vi "UHR-Fleezers Control (fpga) - Leonardo 04-2018 V2.vi"() -> ()   [LabVIEW 2013]
doc: "UHR-Fleezers Instrument Control Code (fpga)"
uses:
  <vilib>/Platform/TimedLoop/XDataNode/timing_clust.ctl
  <vilib>/Platform/TimedLoop/XDataNode/nitl_modes.ctl
  <vilib>/Platform/TimedLoop/XDataNode/wakeup.ctl
  <vilib>/rvi/eio/common/nirviEmuTemplateMethod_errors.vi
  <vilib>/rvi/Emulation/niFpgaSctlEmulationGetInTimedLoop.vi
  <vilib>/rvi/Emulation/niFpgaEmulationReportErrorSimple.vi
  <vilib>/rvi/Emulation/niFpgaGetClockAttributes.vi
  <vilib>/rvi/Emulation/niFpgaCriticalErrorInLSC.vi
  <vilib>/rvi/FIFO/Fifo_Resource/nirvififoEmulationReadFpgaImpl.vi
  <vilib>/rvi/DataTransferAndStorage/Container/Common/niFpgaContainerGetUniqueNameForEmu.vi
  <vilib>/rvi/DataTransferAndStorage/Container/Common/niFpgaContainerExecOnDevCompGetState.vi
  <vilib>/rvi/interface/RandomDataEmulation/nirviRandomDataFPGAFIFO.vi
  <vilib>/rvi/interface/RandomDataEmulation/niFpgaRandomDataHandleErrors.vi
  <vilib>/rvi/eio/common/nirviEmuReportErrorAndStop.vi
  <vilib>/rvi/Emulation/niFpgaProcessEmulError.vi
  <vilib>/rvi/FIFO/Fifo_Resource/nirvififoEmulationWriteFpgaImpl.vi
  <vilib>/Platform/TimedLoop/XDataNode/XDataNode.xnode
  <vilib>/eio/EIOMethodNode/EIOMethodNode.xnode
  <vilib>/eio/EIONode/EIONode.xnode
  <vilib>/rvi/DataTransferAndStorage/Container/XNode/niFpgaContainer.xnode
  <vilib>/rvi/FIFO/Fifo_Resource/nirvififoEmulationRead.vi
  <vilib>/rvi/FIFO/Fifo_Resource/niFpgaFifoEmulationRefIn.vi
  <vilib>/rvi/interface/RandomDataEmulation/nirviRandomDataFpgaReadWriteTemplate.vi
  <vilib>/rvi/FIFO/Fifo_Resource/nirvififoEmulationWrite.vi
  <vilib>/addons/control/pid/fpga.llb/XNode/niFpgaPID.xnode
  <vilib>/Platform/TimedLoop/XDataNode/XDNodeRunTimeDep.lvlib
  <vilib>/rvi/Memory/Memory_Emulation/niFpgaMemoryEmulationRefIn.vi
panel:
  in  "Tab Control 2":T1(tab)
  out "BD1 amplitude 1 out":u16
  out "BD1 amplitude 2 out":u16
  in  "FB output range":cluster{"output low":i16, "output high":i16}={"output low"=0, "output high"=3000}
  in  "FB Gains":T2={"proportional gain (Kc)"=10, "integral gain (Kc*Ts/Ti)"=5, "derivative gain (Kc*Td/Ts)"=0}
  in  "RF synth green feedback max":i16=4000
  in  "RD":bool=TRUE
  in  "Swap F1 and F2":bool
  in  "Scan BD":bool
  in  "Start scan":bool
  in  "OSK Bd 1":bool
  in  "Reset Bd 1":bool
  in  "PMODE":bool=TRUE
  in  "Number Interlace Cycles":u8=2 min=1 max=3
  in  "Interlace Off Parameters":u8=1 min=1 max=3
  in  "Interlace ON/OFF":bool
  out "DIO Relative phase":i16
  in  "Phase count adjustment (DIO)":i16
  in  "+ phase (DIO)":bool
  out "DIO Late Counter":u8
  in  "DIO count 1 (ticks)":u16=400
  in  "DIO count 2 (ticks)":u16=400
  in  "DIO count 3 (ticks)":u16=400
  out "AI2 Y Sum Set 2":i16
  out "AI2 Y Sum Set 1":i16
  in  "FB Setpoint Set 1":i16 min=0 step=1
  in  "FB Reset Set 1":bool
  in  "FB On/Off Set 1":bool
  in  "FB Reset Set 2":bool
  in  "FB On/Off Set 2":bool
  in  "FB Setpoint Set 2":i16 min=0 step=1
  in  "Amp switch delay":u8=5
  in  "RF synth bd controls green":bool
  in  "Phase Trap 2":fxp<+,14,14>
  in  "Phase Trap 1":fxp<+,14,14>
  in  "Phase offset method":u8
  in  "BD 2 Amplitude 1":u16
  in  "BD 1 Amplitude 1":u16
  in  "BD 2 Frequency 1":u64
  in  "BD 1 Frequency 1":u64
  in  "BD 2 Amplitude 2":u16
  in  "BD 1 Amplitude 2":u16
  in  "BD 2 Frequency 2":u64
  in  "BD 1 Frequency 2":u64
  in  "BD 2 Amplitude 3":u16
  in  "BD 1 Amplitude 3":u16
  in  "BD 2 Frequency 3":u64
  in  "BD 1 Frequency 3":u64
  in  "BD 2 Delay (Ticks)":u8 caption="Count(Ticks)"
  in  "Next trap write delay (ticks)":u8 caption="Count(Ticks)"
  out "Random phase generated":fxp<+,14,14>
  in  "RF phase reset before cycles":bool
  in  "Trap 1 osc enable":bool
  in  "N trap osc periods":i16
  in  "Trap osc period (pts)":i16
  in  "Osc traps":bool
  in  "Initiate trap osc":bool
  in  "Ready Write":bool
  in  "Data":i64
  in  "Address 2":u32
  in  "Osc trap cont.":bool
  in  "Trap 2 osc enable":bool
  out "green FB running":bool
  in  "APD 2 AO scale factor":i16=1
  in  "BD 1 Delay (ticks)":u8
  in  "Tab Control":T3(tab)=enum."MCL trap control"
  in  "Set 3":bool
  in  "Set 2":bool=TRUE
  in  "Set 1":bool=TRUE
  in  "Trap Pos to FIFO":bool
  in  "N of AI1 Int Acq Sets":i16=2 min=1 max=3 step=1
  out "AI Late Counter":u8
  in  "ai count":u16=400
  in  "+ phase":bool
  in  "Phase count adjustment":i16
  out "Relative phase":i16
  in  "AI to FIFO":bool
  out "BD1 Frequency Out 1":u64
  out "BD1 Frequency Out 2":u64
  out "Trap Pos FIFO Timeout":u16
  out "Trap AI FIFO Timeout":u16
  in  "Trap FIFO Set Timeout":i32
  in  "Scan freq.  increment":i64
  in  "Scan steps":u64
  in  "Number of scans":u16
  in  "Cycles per step":u64
  in  "Raster setpoint":fxp<+/-,16,1>
  in  "Raster to target force":bool
  out "Actual Scan freq":u64
  in  "Cont. Scan":bool
  out "Scan I":u64
  in  "Abort scan":bool
  out "Scanning":bool
  in  "FB Min frequency":u64
  in  "FB Max Frequency":u64
  in  "Dynamic Force FB (Ronen)":bool
  in  "Trap pos. FB Range":T4={"FB2 output low"=-1.0, "FB2 output high"=0.999969482421875}
  in  "Trap Pos. FB Gains":T5={"proportional gain (Kc)"=0.999969482421875, "integral gain (Kc*Ts/Ti)"=0.999969482421875, "derivative gain (Kc*Td/Ts)"=0.0}
  in  "B factor":fxp<+/-,32,16>
  in  "Negate Diff?":bool
  in  "Diff FB Measurement?":bool
  in  "FB Trig Integrate":u32=1
  out "TTrig?":bool
  in  "TTrig Negate Pos":bool=TRUE
  out "Trap Pos FB Int Signal":fxp<+/-,24,9> format="%.18g"
  out "Trap Pos FB Int-Norm Signal":fxp<+/-,16,1> format="%.16g"
  in  "FPGA TTrig Thresh":i64
  in  "FPGA Trap Trig":bool
  out "Trap Pos FB Action":i64
  in  "Trap Pos. FB Offset Factor":i64
  in  "Trap Pos. FB Mult Factor":i64=2
  in  "Trap Pos. FB Reset":bool
  in  "Trap Pos FB Monitor T1 or T2":bool
  in  "AI1 X Scale":u16
  in  "Trap Pos FB Int Count":u16=100
  in  "Trap Pos FB Negate Action":bool
  out "AI1 X Set 2":fxp<+/-,16,1>
  out "AI1 X Set 1":fxp<+/-,16,1>
  in  "Trap Pos. FB SP":fxp<+/-,16,1>
  in  "Force feedback":bool
  out "TTrig Sig":i64
  out "TTrig Fin Thresh":i64
  in  "1D or 2D Scan?":bool
  in  "Abort scan (MCL)":bool
  in  "MCL Scan Axis":bool
  in  "Cont. Scan (MCL)":bool
  out "Scan I (MCL)":u64
  in  "Number of scans (MCL)":u16
  out "Scanning MCL":bool
  in  "Scan steps (MCL)":u64
  in  "Cycles per step (MCL)":u64
  in  "Scan freq.  increment (MCL)":i16
  in  "Start scan (MCL)":bool
  in  "AO2 (X)":i16
  in  "AO1 (Y)":i16
  out "MCL Late Counter":u8
  in  "MCL count":u32=800
  out "MCL Relative Phase":i16
  in  "Phase count adjustment (MCL)":i16
  in  "+ phase (MCL)":bool
  in  "Lifetime events to read blue":u16=100
  in  "Lifetime read blue fifo":bool
  out "lifetime events in fifo":u16
  out "APD2 int gate":bool
  in  "APD Gate Operating Mode":u8 max=2 step=1
  in  "Invert APD Gate":bool
  in  "APD Gate OFF Count":u16=100
  in  "APD Gate ON Count":u16=300
  out "APD 1 Gate Late Counter":u8
  out "APD 1 Gate Relative Phase":i16
  in  "Phase count adjustment (APD 1 Gate)":i16
  in  "+ phase (APD 1 Gate)":bool
  out "APD 2 Counts 0":u32
  out "APD 2 Counts 1":u32
  out "APD 1 Counts 0":u32
  out "APD 1 Counts 1":u32
  in  "Phase count adjustment (APD 2 Gate)":i16
  out "APD 2 Gate Late Counter":u8
  out "APD 2 Gate Relative Phase":i16
  in  "+ phase (APD 2 Gate)":bool
  out "APD 3 Counts 0":u32
  out "APD 3 Counts 1":u32
  out "APD 3 Gate Late Counter":u8
  in  "Phase count adjustment (APD 3 Gate)":i16
  out "APD 3 Gate Relative Phase":i16
  in  "+ phase (APD 3 Gate)":bool
  out "APD1 int gate":bool
  out "APD3 int gate":bool
  in  "Lifetime timeout APD1":u16=200
  in  "APD to FIFO":bool
  in  "APD Acq Rate Count":u32=20000000
  out "APD Acq Late Counter":u16
  out "APD Acq Relative Phase":i16
  in  "+ phase (APD Acq)":bool
  in  "Phase Count Adjustment (APD Acq)":i16
  in  "APD 1 AO scale factor":i16=1
  out "APD2 out state":bool
  out "APD1 out state":bool
  out "APD Acq Late?":bool
  in  "D3 2":i16
  in  "I3 2":i16=5
  in  "P3 2":i16=10
  in  "Green FB Setpoint 2":i16=250 min=0 step=1
  in  "Green FB Reset 2":bool
  in  "Green Filter Flipper":bool
  in  "Green interlace OFF count":u16=100
  out "GI Relative phase":i16
  in  "Phase count adjustment (GI)":i16
  in  "+ phase (GI)":bool
  in  "Green interlace ON count":u16=300
  out "GI Late Counter":u8
  in  "Invert GI":bool
  in  "Operating Mode":u8 max=2 step=1
  in  "Current Out":u16=30000
  in  "Green int current ON count adj":u32=150
  in  "Green interlace OFF count 2":u32=900
  in  "Green interlace ON count 2":u32=300
  out "GI Late Counter 2":u16
  in  "Green FB Count":u32=1200
  in  "Phase count adjustment (GI) 2":i16=20
  in  "Green FB Setpoint":i16=250 min=0 step=1
  in  "Invert GI 2":bool
  out "GI Relative phase 2":i16
  in  "+ phase (GI) 2":bool
  in  "Phase count adjustment (Green FB)":i16=10
  out "Green Late Counter":u16
  out "Green FB Relative Phase":i16
  in  "+ phase (Green FB)":bool
  out "Green FB Signals":T6
  out "Green FB Sum":i16
  in  "Green FB Gains":T2={"proportional gain (Kc)"=10, "integral gain (Kc*Ts/Ti)"=5, "derivative gain (Kc*Td/Ts)"=0}
  in  "Green FB On/Off":bool
  in  "Green FB Reset":bool
  out "Green FB Late?":bool
  out "GI Late?":bool
  in  "Operating Mode 2":u8=2 max=2 step=1
  in  "Chassis2/Mod4/AO1":u16
  in  "+ phase (RI)":bool
  out "RI Relative phase":i16
  out "RI Late Counter":u8
  in  "Red interlace ON count":u16=300
  in  "Red interlace OFF count":u16=100
  in  "Invert RI":bool
  in  "Red Laser Operating Mode":u8 max=2 step=1
  in  "Phase count adjustment (RI)":i16
  in  "Phase count adjustment (BI D)":i16
  in  "Blue Laser Operating Mode (D)":u8 max=2 step=1
  in  "Invert BI (D)":bool
  in  "Blue interlace OFF count (D)":u16=100
  in  "Blue interlace ON count (D)":u16=300
  out "Blue Late Counter (D)":u8
  out "BI Relative phase (D)":i16
  in  "+ phase (BI D)":bool
  in  "Lifetime to FIFO":bool
  out "lifetime (ticks)":u16
  # "Raster Scan AOD"
  # "1 (X)"
  # "2 (Y)"
  # "IR Intensity Feedback (RF BD 1)"
  # "FB Gains Set 1"
  # "FB output range 1"
  # "IR Intensity Feedback (RF BD 2) -\nonly when using BD 2 for green laser AOM (not trap Y)"
  # "Keep below 4096 (12 bits) to stay within range of RF board. Going over doesn't saturate, it truncates higher bits."
  # "RF phase offset control"
  # "Methods are:\n0 - Default, do nothing at all (no phase offset writes)\n1 - Manual phase adjustment\n2 - Cycle the phase adjustment using the input phase numbers as increment values for each cycle"
  # "False is usual, True is external loop method"
  # "Parameters if using the external RF switching loop"
  # "Parameters if using the usual internal RF switching method"
  # "FB Triggering Excitation Laser"
  # "Trap Pos. FB Gains"
  # "Trap Pos. FB Range"
  # "AO1 (Y)"
  # "2D"
  # "Trap 3"
  # "1D"
  # "AO2 (X)"
  # "Fl Laser"
  # "APD AO for aligning"
  # "Detection Loop"
  # "Green fluorescent laser digital gate interlacing loop"
  # "0 Forced ON\n1 Forced OFF\n2 Interlacing"
  # "ALEX settings:"
  # "Controls for usual IA ME controls green AOM"
  # "Controls for RF synth board controls green AOM"
  # "Green FB Gains"
  # "Red fluorescent laser digital gate interlacing loop"
  # "Detection Loop"
  # "0 Forced ON\n1 Forced OFF\n2 Interlacing"
  # "Analog/FB Control Loop\n(Disabled)"
  # "Digital Control Loop"
  # "Blue laser intensity reading"
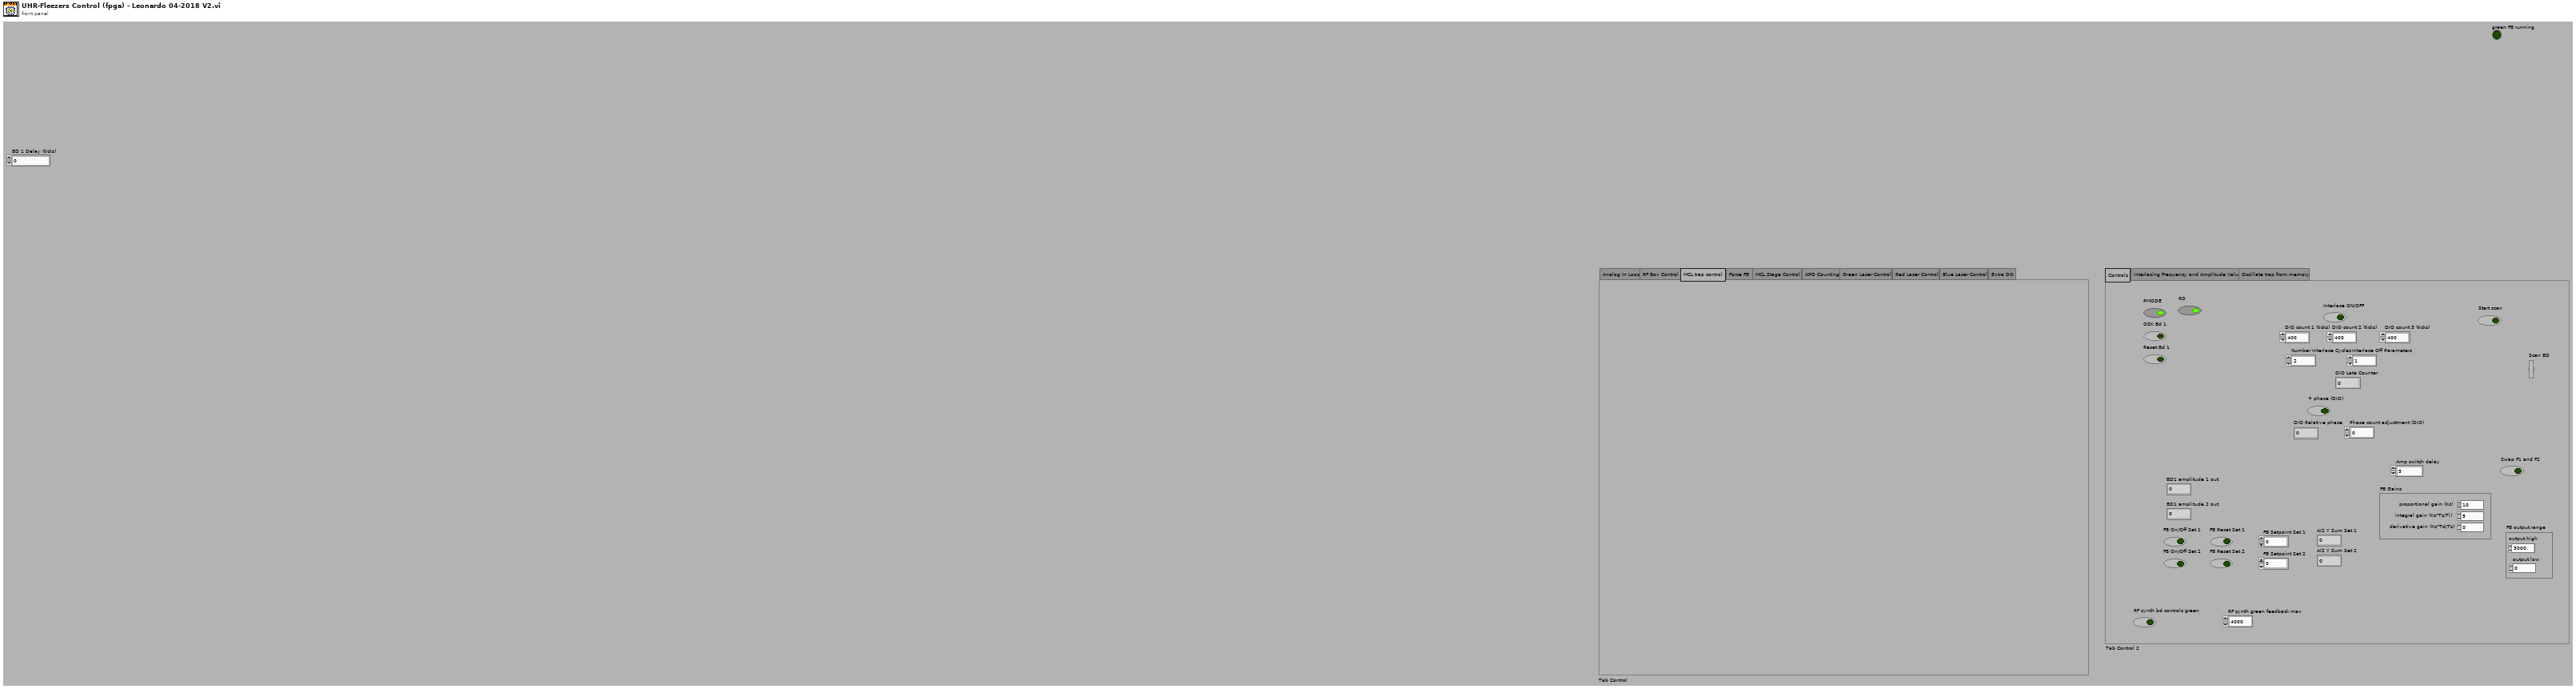
[diagram p1: front panel]
types:
  T1 = enum32{"Controls", "Interlacing Frequency and Amplitude Values", "Oscillate trap from memory"}
  T2 = cluster{"proportional gain (Kc)":i16, "integral gain (Kc*Ts/Ti)":i16, "derivative gain (Kc*Td/Ts)":i16}
  T3 = enum32{"Analog In Loop", "RF Box Control", "MCL trap control", "Force FB", "MCL Stage Control", "APD Counting", "Green Laser Control", "Red Laser Control", "Blue Laser Control", "Extra DO"}
  T4 = cluster{"FB2 output low":fxp<+/-,16,1>, "FB2 output high":fxp<+/-,16,1>}
  T5 = cluster{"proportional gain (Kc)":fxp<+/-,16,1>, "integral gain (Kc*Ts/Ti)":fxp<+/-,16,1>, "derivative gain (Kc*Td/Ts)":fxp<+/-,16,1>}
  T6 = cluster{"Green FB Ch 0":i16, "Green FB Ch 1":i16, "Green FB Ch 2":i16}
  T7 = typedef "XDNodeRunTimeDep.lvlib/timing_clust.ctl" = cluster{"Expected End [f-1]":u64, "Actual End [f-1]":u64, "Finished Late? [f-1]":bool, "Expected End [i-1]":u64, "Actual End [i-1]":u64, "Finished Late? [i-1]":bool, "Expected Start [i]":u64, "Actual Start [i]":u64, "Expected Start [f]":u64, "Actual Start [f]":u64, "Source Name":string, "Structure Name":string, "Period":i64, "Deadline":i64, "Offset":i64, "Start":i64, "Priority":i32, "Timeout":i32, "Mode":T8, "Wakeup Reason":T9, "Error":errorcluster, "Source Type":string, "Secondary Source Type":string, "Global End Time":u64, "Global Start Time":u64, "Frame Duration":u64, "Iteration Duration":u64, "Assigned CPU":i32, "I/O Scan Engine Mode":u32}
  T8 = typedef "XDNodeRunTimeDep.lvlib/nitl_modes.ctl" = enum32{"No Change", "Process missed periods, maintain original phase", "Discard missed periods, maintain original phase", "Process missed periods, ignore original phase", "Discard missed periods, ignore original phase"}
  T9 = typedef "XDNodeRunTimeDep.lvlib/wakeup.ctl" = enum32{"Normal", "Aborted", "Asynchronous wakeup", "Timing source error", "Timed loop error", "Timeout"}
  T10 = cluster{"Chassis2/Mod2/AI0":i16, "Chassis2/Mod2/AI1":i16, "Chassis2/Mod2/AI2":i16}
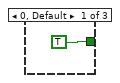
[diagram p3: hidden frame]
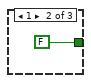
[diagram p4: hidden frame]
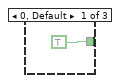
[diagram p8: hidden frame]
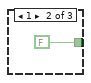
[diagram p9: hidden frame]
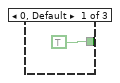
[diagram p10: hidden frame]
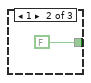
[diagram p11: hidden frame]
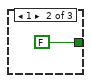
[diagram p13: hidden frame]
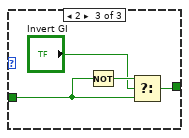
[diagram p14: hidden frame]
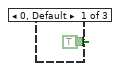
[diagram p15: hidden frame]
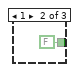
[diagram p16: hidden frame]
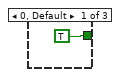
[diagram p18: hidden frame]
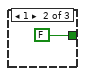
[diagram p19: hidden frame]
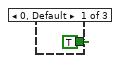
[diagram p20: hidden frame]
diagram:
  w3 = FALSE
  w4 = FALSE
  # "BD2 amp"
  # "BD1 amp"
  # "BD2 amp"
  # "BD1 amp"
  # "timing array current index"
  # "timing array"
  # "timing counter (phase adjusted here)"
  # "late counter"
  n1 = while {
    stop <- FALSE stop-if-true
    n2 = xnode "FPGA I/O Node"("Connector0/DIO3"="Green Filter Flipper", "Chassis2/Mod1/AO1"="Chassis2/Mod4/AO1") -> ()  [unwired: 2 in, 2 out]
    n3 = call "Loop Timer11"("Count(Ticks)"=u32 40000 ("Extra DO Counts")) -> ()  [unwired: 1 out]
  }
  n4 = disable-structure shown="Disabled" {
    frame Disabled {
      w18 = i16 2 items=["UnSet Ready", "ReadWrite", "Wait Ready"]
      n5 = while "Handshake memory transfer for trap oscillation sin wave data" {
        shift-right: [w20] -> _
        shift-left: w18 -> [w21]
        stop <- FALSE stop-if-true
        # "Write"
        n6 = case shown="1" w21 {
          tunnel: [w24 w29 w30] -> w20
          frame 3, Default {
            w22 = i16 2 items=["UnSet Ready", "ReadWrite", "Wait Ready"]
            w23 = i16 1 items=["UnSet Ready", "ReadWrite", "Wait Ready"]
            n7 = Select(t=w23, s="Ready Write", f=w22) -> (s? t:f=w24:i16)
          }
          frame 1 {
            w29 = i16 0 items=["UnSet Ready", "ReadWrite", "Wait Ready"]
            n8 = xnode ("Memory Write")("Address"="Address 2", "Data"="Data", "Memory In"=refnum<k21> "Trap osc memory") -> ()  [unwired: 1 out]
          }
          frame 0 {
            w30 = i16 2 items=["UnSet Ready", "ReadWrite", "Wait Ready"]
            n9 = local write "Ready Write"(FALSE ("Ready Read")) -> ()
          }
        }
      }
    }
    frame Enabled {
    }
  }
  n10 = flat-sequence "FPGA initialization to do before running any of the loops" {
    tunnel: [u16 0 ("DIO count 3 (ticks)")] -> w2
    tunnel: [w39] -> _
    frame #0 {
      # "UDCLK out enable and set low"
      # "WR"
      # "BD 2"
      # "BD 1"
      # "With the RF synth board initialization now done in a separate fpga vi, now when this vi is started, board is already configured and is ready for interlacing. Just need to set WR high and enabled UDCLK as write and set to low.\nbefore setting data and address bits."
      # "Start up expansion chassis early\nto avoid delays later"
      # "Set data and address values to something safe (a correct setting) so any initial WR and udclk flipping doesn't have a chance to mess anything up. Safe would be setting an unused data entry:"
      n11 = xnode "FPGA I/O Method Node"("Enable"=TRUE) -> ("FPGA I/O Out"=w33:refnum<k21>)  [unwired: 1 in]
      n12 = xnode "FPGA I/O Method Node"("Enable"=TRUE) -> ("FPGA I/O Out"=w36:refnum<k21>)  [unwired: 1 in]
      n13 = xnode "FPGA I/O Node"("Chassis2/Mod1/AO0"=u16 0 ("Chassis2/Mod4/AO0")) -> ("Chassis2/Mod2/AI0"=w39:i16)  [unwired: 2 in, 2 out]
      n14 = xnode "FPGA I/O Node"("Connector1/DIO15"=TRUE) -> ()  [unwired: 1 in, 1 out]
      n15 = xnode "FPGA I/O Node"("I/O Item"=FALSE ("Connector1/DIO30"), "FPGA I/O In"=w33) -> ()  [unwired: 1 out]
      n16 = xnode "FPGA I/O Node"("I/O Item"=FALSE ("Connector1/DIO30"), "FPGA I/O In"=w36) -> ()  [unwired: 1 out]
      n17 = xnode "FPGA I/O Node"("Connector1/DIO0"=FALSE, "Connector1/DIO1"=FALSE, "Connector1/DIO2"=FALSE, "Connector1/DIO3"=FALSE, "Connector1/DIO4"=FALSE, "Connector1/DIO5"=FALSE, "Connector1/DIO6"=FALSE, "Connector1/DIO7"=FALSE, "Connector1/DIO8"=FALSE, "Connector1/DIO9"=FALSE, "Connector1/DIO10"=FALSE, "Connector1/DIO11"=FALSE, "Connector1/DIO12"=FALSE, "Connector1/DIO13"=FALSE, "Connector1/DIO20"=FALSE, "Connector1/DIO21"=FALSE, "Connector1/DIO22"=FALSE, "Connector1/DIO23"=FALSE, "Connector1/DIO24"=FALSE, "Connector1/DIO25"=FALSE, "Connector1/DIO26"=FALSE, "Connector1/DIO27"=FALSE, "Connector1/DIO14"=FALSE) -> ()  [unwired: 23 in, 23 out]
    }
  }
  n18 = node-c288() -> (w10:T7)  [unwired: 1 in]
  n19 = timed-loop "RF box board DIO control: control bits" {
    timing: w10 -> [_]
    timing-out: [_] -> w9
    tunnel: [w66] -> _
    tunnel: w2 -> [w66]
    stop <- FALSE stop-if-true
    n20 = xnode "FPGA I/O Node"("Connector1/DIO16"="RD", "Connector1/DIO17"="PMODE", "Connector1/DIO18"="OSK Bd 1", "Connector1/DIO19"="Reset Bd 1") -> ()  [unwired: 4 in, 4 out]
  }
  n21 = node-c288(w9) -> ()
  n22 = local read "AO1 (Y)"() -> (w12:i16)
  n23 = local read "AO2 (X)"() -> (w11:i16)
  n24 = To Unsigned Long Integer(number=w2) -> (unsigned 32bit integer=w5:u32)
  n25 = while "DAQ AI set 1" {
    shift-right: [w73] -> _
    shift-left: w2 -> [w78]
    stop <- FALSE stop-if-true
    n26 = flat-sequence {
      tunnel: w78 -> [w89]
      tunnel: [w88] -> w76
      tunnel: [w89] -> w75
      tunnel: [w99] -> w86
      tunnel: [w98] -> w85
      tunnel: [w97] -> w84
      tunnel: [w96] -> w83
      tunnel: [w95] -> w82
      tunnel: [w94] -> w81
      tunnel: [w93] -> w80
      tunnel: [w92] -> w79
      tunnel: [w91] -> w77
      tunnel: w76 -> [w91]
      tunnel: w75 -> [w90]
      tunnel: [w90] -> w74
      tunnel: [w129] -> w73
      tunnel: w86 -> [w155]
      tunnel: w85 -> [w121]
      tunnel: w84 -> [w122]
      tunnel: w83 -> [w101]
      tunnel: w82 -> [w145]
      tunnel: w81 -> [w144]
      tunnel: w80 -> [w143]
      tunnel: w79 -> [w142]
      tunnel: w77 -> [w139]
      tunnel: w74 -> [w136]
      frame #0 {
        n27 = call "Loop Timer"("Count(Ticks)"=w89) -> ("Tick Count(Ticks)"=w88:u32)
      }
      frame #1 {
        n28 = xnode "FPGA I/O Node"("Connector1/DIO31"=TRUE ("Connector1/DIO33")) -> ("Connector0/AI0"=w99:i16, "Connector0/AI1"=w98:i16, "Connector0/AI2"=w97:i16, "Connector0/AI3"=w96:i16, "Connector0/AI4"=w95:i16, "Connector0/AI5"=w94:i16, "Connector0/AI6"=w93:i16, "Connector0/AI7"=w92:i16)  [unwired: 9 in, 9 out]
      }
      frame #2 {
        w125 = FALSE ("AI to FIFO")
        # "Normalize by trap bead QPD sum, AI3"
        # "Adjust phase after data acquired if button pressed"
        n29 = feedback #1(i16 1) -> (w148:i16)
        n30 = Increment(x=w148) -> (x+1=w154:i16)
        n31 = Scale By Power Of 2(n="AI1 X Scale", x=w121) -> (x*2^n=w119:i16)
        n32 = Greater?(x=w154, y="N of AI1 Int Acq Sets") -> (0:w151:bool)
        n33 = Select(t=i16 1, s=w151, f=w154) -> (s? t:f=w153:i16)
        n34 = feedback-in #1(w153) -> ()
        n35 = Divide(x=w119, y=w101) -> (x/y=w118:fxp<+/-,16,1>)
        n36 = feedback #2(w125) -> (w123:bool)
        n37 = feedback #3(w125) -> (w141:bool)
        n38 = case shown="1, Default" w148 {
          tunnel: w122 -> [w178 w185 _]
          tunnel: ["Set 1" "Set 2" "Set 3"] -> w146
          tunnel: ["AI to FIFO" w187 w192] -> w140
          tunnel: w141 -> [_ w187 w192]
          tunnel: ["Trap Pos to FIFO" w186 w191] -> w124
          tunnel: w123 -> [_ w186 w191]
          tunnel: w118 -> [w177 w184 _]
          tunnel: [w176 w182 FALSE] -> w105
          tunnel: [w175 w183 u64 0 ("BD1 Frequency Out 2")] -> w104
          frame 1, Default {
            n39 = local read "BD1 Frequency Out 1"() -> (w175:u64)
            n40 = Compound Arithmetic op=AND("Trap Pos to FIFO", "Set 1", "AI to FIFO") -> (w176:bool)
            "AI2 Y Sum Set 1" <- w178
            "AI1 X Set 1" <- w177
          }
          frame 2 {
            n41 = local read "BD1 Frequency Out 2"() -> (w183:u64)
            n42 = Compound Arithmetic op=AND(w186, "Set 2", w187) -> (w182:bool)
            "AI2 Y Sum Set 2" <- w185
            "AI1 X Set 2" <- w184
          }
          frame 3 {
          }
        }
        n43 = And(x=w146, y=w140) -> (x .and. y?=w147:bool)
        n44 = case shown="True" w147 {
          tunnel: w155 -> [_ w206]
          tunnel: w121 -> [_ w205]
          tunnel: w122 -> [_ w204]
          tunnel: w101 -> [_ w203]
          tunnel: w145 -> [_ w202]
          tunnel: w144 -> [_ w201]
          tunnel: w143 -> [_ w200]
          tunnel: w142 -> [_ w199]
          tunnel: 0 ("DMA buffer timeout") -> [_ w208]
          frame False {
          }
          frame True {
            n45 = Build Array(w206, w205, w204, w203, w202, w201, w200, w199) -> (w207:i16[])
            n46 = for {
              tunnel: w207 -> [w210] mode=indexing
              tunnel: w208 -> [w211]
              tunnel: [w209] -> w197 mode=indexing
              n47 = xnode ("FIFO Write")("Element"=w210, "Timeout"=w211) -> ("Timed Out?"=w209:bool)  [unwired: 1 in, 1 out]
            }
            n48 = Or Array Elements(Boolean array=w197) -> (logical OR=w194:bool)
            n49 = Boolean To (0,1)(Boolean=w194) -> (0, 1=w196:i16)
            n50 = feedback #4(u16 0) -> (w195:u16)
            n51 = Add(x=w196, y=w195) -> (x+y=w193:u16)
            "Trap AI FIFO Timeout" <- w193
            n52 = feedback-in #4(w193) -> ()
          }
        }
        n53 = feedback-in #2(w124) -> ()
        n54 = feedback-in #3(w140) -> ()
        n55 = case shown="True" w105 {
          tunnel: w104 -> [_ w161]
          tunnel: [u8 0 w158] -> w103
          frame False {
          }
          frame True {
            n56 = Split Number(x=w161) -> (hi(x)=w162:u32, lo(x)=w163:u32)
            n57 = Split Number(x=w162) -> (lo(x)=w164:u16)  [unwired: 1 out]
            n58 = Split Number(x=w163) -> (hi(x)=w165:u16, lo(x)=w166:u16)
            n59 = Build Array "BD 1 nu Stack"(w164, w165, w166) -> (w160:u16[])
            n60 = for {
              tunnel: w160 -> [w173] mode=indexing
              shift-right: [w169] -> w158
              shift-left: u8 0 -> [w170]
              n61 = xnode ("FIFO Method Node")("Element"=w173, "Timeout"="Trap FIFO Set Timeout") -> ("Timed Out?"=w172:bool)  [unwired: 1 in, 1 out]
              n62 = Boolean To (0,1)(Boolean=w172) -> (0, 1=w171:i16)
              n63 = To Unsigned Byte Integer(number=w171) -> (unsigned 8bit integer=w168:u8)
              n64 = Add(x=w168, y=w170) -> (x+y=w169:u8)
            }
          }
        }
        n65 = To Unsigned Word Integer(number=w103) -> (unsigned 16bit integer=w102:u16)
        n66 = feedback #5(u16 0) -> (w116:u16)
        n67 = Add(x=w102, y=w116) -> (x+y=w115:u16)
        "Trap Pos FIFO Timeout" <- w115
        n68 = feedback-in #5(w115) -> ()
        n69 = feedback-in #6(w139) -> ()
        n70 = feedback #6(w139) -> (w138:u32)
        n71 = Subtract(x=w139, y=w138) -> (x-y=w137:u32)
        n72 = xnode "FPGA I/O Node"("Connector1/DIO31"=FALSE ("Connector1/DIO34")) -> ()  [unwired: 1 in, 1 out]
        n73 = Subtract(x=w137, y=w136) -> (x-y=w107:u32)
        n74 = Boolean To (0,1)(Boolean="+ phase") -> (0, 1=w132:i16)
        n75 = Multiply(x=w132, y="Phase count adjustment") -> (x*y=w126:i16)
        n76 = Subtract(x="ai count", y=w107) -> (x-y=w130:u32)
        n77 = Number To Boolean Array(number=w107) -> (Boolean array=w108:bool[])
        n78 = feedback #7(i16 0) -> (w128:i16)
        n79 = Add(x=w130, y=w126) -> (x+y=w129:u32)
        n80 = Subtract(x=w128, y=w126) -> (x-y=w127:i16)
        "Relative phase" <- w127
        n81 = feedback-in #7(w127) -> ()
        n82 = Or Array Elements(Boolean array=w108) -> (logical OR=w106:bool)
        n83 = Boolean To (0,1)(Boolean=w106) -> (0, 1=w113:i16)
        n84 = To Unsigned Byte Integer(number=w113) -> (unsigned 8bit integer=w110:u8)
        n85 = feedback #8(u8 0) -> (w111:u8)
        n86 = Add(x=w110, y=w111) -> (x+y=w109:u8)
        "AI Late Counter" <- w109
        n87 = feedback-in #8(w109) -> ()
      }
    }
  }
  n88 = while "MCL stage control" {
    shift-right: [w224] -> _
    shift-left: w2 -> [w227]
    shift-right: [w217] -> _
    shift-left: w12 -> [w214]
    shift-right: [w216] -> _
    shift-left: w11 -> [w212]
    stop <- FALSE stop-if-true
    n89 = flat-sequence {
      tunnel: w227 -> [w230]
      tunnel: [w229] -> w223
      tunnel: [w230] -> w221
      tunnel: [w232] -> w215
      tunnel: w214 -> [w232]
      tunnel: [w231] -> w213
      tunnel: w212 -> [w231]
      tunnel: w223 -> [w236]
      tunnel: [w236] -> w222
      tunnel: w221 -> [w235]
      tunnel: [w235] -> w220
      tunnel: w215 -> [w234]
      tunnel: w213 -> [w233]
      tunnel: w222 -> [w244]
      tunnel: w220 -> [w243]
      tunnel: [w244] -> w226
      tunnel: [w243] -> w225
      tunnel: [w242] -> w219
      tunnel: [w241] -> w218
      tunnel: [w316] -> w224
      tunnel: w226 -> [w323]
      tunnel: w225 -> [w320]
      tunnel: w219 -> [w318]
      tunnel: w218 -> [w317]
      tunnel: [w318] -> w217
      tunnel: [w317] -> w216
      frame #0 {
        n90 = call "Loop Timer3"("Count(Ticks)"=w230) -> ("Tick Count(Ticks)"=w229:u32)
      }
      frame #1 {
        n91 = xnode "FPGA I/O Node"("Connector0/AO1"=w234, "Connector0/AO2"=w233) -> ()  [unwired: 2 in, 2 out]
      }
      frame #2 {
        n92 = local read "Scanning MCL"() -> (w256:bool)
        n93 = Or(x=w256, y="Start scan (MCL)") -> (x .or. y?=w251:bool)
        n94 = Not(x="Abort scan (MCL)") -> (.not. x?=w249:bool)
        n95 = And(x=w249, y=w251) -> (x .and. y?=w248:bool)
        n96 = case "Raster scan" shown="False" w248 {
          tunnel: [w257 w300] -> w253
          tunnel: "Start scan (MCL)" -> [_ w285]
          tunnel: [w257 w261] -> w237
          frame False {
            w257 = i16 0
            n97 = local write "Scanning MCL"(FALSE ("scanning")) -> ()
          }
          frame True {
            w271 = i16 0
            w270 = u64 0
            # "scan incr."
            # "freq. incr. mult."
            # "count steps"
            # "count number of cycles"
            n98 = feedback #9(w270) -> (w297:u64)
            n99 = Select(t=w270, s=w285, f=w297) -> (s? t:f=w299:u64)
            n100 = Increment(x=w299) -> (x+1=w296:u64)
            n101 = Greater?(x="Cycles per step (MCL)", y=w296) -> (0:w280:bool)
            n102 = Select(t=w296, s=w280, f=w270) -> (s? t:f=w295:u64)
            n103 = feedback-in #9(w295) -> ()
            n104 = feedback #10(w270) -> (w294:u64)
            n105 = Select(t=w270, s=w285, f=w294) -> (s? t:f=w289:u64)
            n106 = Increment(x=w289) -> (x+1=w293:u64)
            n107 = Add(x="Scan steps (MCL)", y="Scan steps (MCL)") -> (x+y=w292:u64)
            n108 = Select(t=w289, s=w280, f=w293) -> (s? t:f=w275:u64)
            n109 = Greater?(x=w292, y=w275) -> (0:w274:bool)
            n110 = Select(t=w275, s=w274, f=w270) -> (s? t:f=w290:u64)
            n111 = feedback-in #10(w290) -> ()
            n112 = Equal?(x="Scan steps (MCL)", y=w275) -> (x = y?=w279:bool)
            n113 = Greater?(x="Scan steps (MCL)", y=w289) -> (0:w288:bool)
            n114 = feedback #11(w271) -> (w291:i16)
            n115 = Select(t=w271, s=w285, f=w291) -> (s? t:f=w277:i16)
            n116 = Increment(x=w277) -> (x+1=w287:i16)
            n117 = Decrement(x=w277) -> (x-1=w286:i16)
            n118 = Select(t=w287, s=w288, f=w286) -> (s? t:f=w278:i16)
            n119 = Select(t=w277, s=w279, f=w278) -> (s? t:f=w276:i16)
            n120 = Select(t=w277, s=w280, f=w276) -> (s? t:f=w272:i16)
            n121 = Select(t=w272, s=w274, f=w271) -> (s? t:f=w273:i16)
            n122 = feedback-in #11(w273) -> ()
            n123 = feedback #12(w270) -> (w284:u64)
            n124 = Select(t=w270, s=w285, f=w284) -> (s? t:f=w259:u64)
            n125 = Increment(x=w259) -> (x+1=w281:u64)
            n126 = Select(t=w259, s=w274, f=w281) -> (s? t:f=w260:u64)
            n127 = Greater?(x="Number of scans (MCL)", y=w260) -> (0:w267:bool)
            n128 = Multiply(x="Scan freq.  increment (MCL)", y=w277) -> (x*y=w300:i16)
            n129 = Select(t=TRUE, s="Cont. Scan (MCL)", f=w267) -> (s? t:f=w266:bool)
            "Scanning MCL" <- w266
            n130 = Select(t=w260, s=w266, f=w270) -> (s? t:f=w282:u64)
            n131 = feedback-in #12(w282) -> ()
            n132 = Increment(x=w260) -> (x+1=→"Scan I (MCL)":u64)
            n133 = To Word Integer(number=w259) -> (16bit integer=w262:i16)
            n134 = Multiply(x=w262, y="Scan freq.  increment (MCL)") -> (x*y=w261:i16)
          }
        }
        n135 = Select(t=w237, s="1D or 2D Scan?", f=i16 0) -> (s? t:f=w238:i16)
        n136 = Select(t=w253, s="MCL Scan Axis", f=w238) -> (s? t:f=w254:i16)
        n137 = Select(t=w238, s="MCL Scan Axis", f=w253) -> (s? t:f=w252:i16)
        n138 = Add(x="AO2 (X)", y=w252) -> (x+y=w241:i16)
        n139 = Add(x="AO1 (Y)", y=w254) -> (x+y=w242:i16)
      }
      frame #3 {
        n140 = feedback-in #13(w323) -> ()
        n141 = feedback #13(w323) -> (w322:u32)
        n142 = Boolean To (0,1)(Boolean="+ phase (MCL)") -> (0, 1=w314:i16)
        n143 = Subtract(x=w323, y=w322) -> (x-y=w321:u32)
        n144 = Multiply(x=w314, y="Phase count adjustment (MCL)") -> (x*y=w310:i16)
        n145 = Subtract(x=w321, y=w320) -> (x-y=w302:u32)
        n146 = Subtract(x="MCL count", y=w302) -> (x-y=w312:u32)
        n147 = feedback #14(i16 0) -> (w311:i16)
        n148 = Subtract(x=w311, y=w310) -> (x-y=w309:i16)
        "MCL Relative Phase" <- w309
        n149 = feedback-in #14(w309) -> ()
        n150 = Number To Boolean Array(number=w302) -> (Boolean array=w303:bool[])
        n151 = Or Array Elements(Boolean array=w303) -> (logical OR=w301:bool)
        n152 = Boolean To (0,1)(Boolean=w301) -> (0, 1=w308:i16)
        n153 = Add(x=w312, y=w310) -> (x+y=w316:u32)
        n154 = To Unsigned Byte Integer(number=w308) -> (unsigned 8bit integer=w305:u8)
        n155 = feedback #15(u8 0) -> (w306:u8)
        n156 = Add(x=w305, y=w306) -> (x+y=w304:u8)
        "MCL Late Counter" <- w304
        n157 = feedback-in #15(w304) -> ()
      }
    }
  }
  n158 = while "APD 2 Counter" {
    tunnel: w2 -> [_]
    stop <- FALSE stop-if-true
    n159 = flat-sequence {
      frame #0 {
        n160 = xnode "FPGA I/O Method Node"("FPGA I/O In"=refnum<k21> "Connector0/DIO1" ("APD 2 DO"), "Timeout"=-1) -> ()  [unwired: 2 out]
      }
      frame #1 {
        n161 = local read "APD2 int gate"() -> (w328:bool)
        n162 = case shown="True" w328 {
          frame False {
          }
          frame True {
            n163 = local read "APD2 out state"() -> (w329:bool)
            n164 = case shown="True" w329 {
              frame False {
                n165 = local read "APD 2 Counts 0"() -> (w331:u32)
                n166 = Increment(x=w331) -> (x+1=→"APD 2 Counts 0":u32)
              }
              frame True {
                n167 = local read "APD 2 Counts 1"() -> (w333:u32)
                n168 = Increment(x=w333) -> (x+1=→"APD 2 Counts 1":u32)
              }
            }
          }
        }
      }
    }
  }
  n169 = while "Green fluorescent laser interlacing (Current to IA 532 nm AOM ME amp)." {
    shift-right: [w339] -> _
    shift-left: w2 -> [w342]
    shift-right: [w336] -> _
    shift-left: i16 0 -> [w334]
    stop <- FALSE stop-if-true
    n170 = flat-sequence {
      tunnel: w342 -> [w345]
      tunnel: [w346] -> w341
      tunnel: [w345] -> w340
      tunnel: [w344] -> w335
      tunnel: w334 -> [w344]
      tunnel: [w349] -> w338
      tunnel: w341 -> [w349]
      tunnel: [w348] -> w337
      tunnel: w340 -> [w348]
      tunnel: w335 -> [w347]
      tunnel: [w362] -> w339
      tunnel: [w378] -> w336
      tunnel: w338 -> [w391]
      tunnel: w337 -> [w388]
      frame #0 {
        n171 = call "Loop Timer10"("Count(Ticks)"=w345) -> ("Tick Count(Ticks)"=w346:u32)
      }
      frame #1 {
        n172 = xnode "FPGA I/O Node"("Chassis2/Mod1/AO0"=w347) -> ()  [unwired: 1 in, 1 out]
      }
      frame #2 {
        n173 = local read "RF synth bd controls green"() -> (w353:bool)
        n174 = Subtract(x="Green interlace OFF count 2", y="Green int current ON count adj") -> (x-y=w371:u32)
        n175 = feedback-in #16(w391) -> ()
        n176 = feedback #16(w391) -> (w390:u32)
        n177 = Add(x="Green int current ON count adj", y="Green interlace ON count 2") -> (x+y=w372:u32)
        n178 = Subtract(x=w391, y=w390) -> (x-y=w389:u32)
        n179 = Subtract(x=w389, y=w388) -> (x-y=w355:u32)
        n180 = Not(x=w353) -> (.not. x?=w351:bool)
        n181 = Number To Boolean Array(number=w355) -> (Boolean array=w356:bool[])
        n182 = Boolean To (0,1)(Boolean="+ phase (GI) 2") -> (0, 1=w368:i16)
        n183 = Or Array Elements(Boolean array=w356) -> (logical OR=w354:bool)
        "GI Late?" <- w354
        n184 = Boolean To (0,1)(Boolean=w354) -> (0, 1=w361:i16)
        n185 = Multiply(x=w368, y="Phase count adjustment (GI) 2") -> (x*y=w364:i16)
        n186 = To Unsigned Word Integer(number=w361) -> (unsigned 16bit integer=w357:u16)
        n187 = feedback #17(u16 0) -> (w359:u16)
        n188 = Add(x=w357, y=w359) -> (x+y=w358:u16)
        "GI Late Counter 2" <- w358
        n189 = feedback-in #17(w358) -> ()
        n190 = feedback #18(i16 0) -> (w365:i16)
        n191 = Subtract(x=w365, y=w364) -> (x-y=w363:i16)
        "GI Relative phase 2" <- w363
        n192 = feedback-in #18(w363) -> ()
        n193 = feedback #19(TRUE) -> (w383:bool)
        n194 = case shown="2" "Operating Mode 2" {
          tunnel: [TRUE FALSE w408] -> w373
          tunnel: w383 -> [_ _ w405]
          frame 0, Default {
          }
          frame 1 {
          }
          frame 2 {
            n195 = Not(x=w405) -> (.not. x?=w407:bool)
            n196 = Select(t=w407, s="Invert GI 2", f=w405) -> (s? t:f=w408:bool)
          }
        }
        n197 = And(x=w373, y="Green FB On/Off") -> (x .and. y?=w352:bool)
        "green FB running" <- w352
        n198 = And(x=w352, y=w351) -> (x .and. y?=w350:bool)
        n199 = case shown="True" w350 {
          tunnel: "Current Out" -> [w392 _]
          tunnel: [w392 w397] -> w377
          frame False {
          }
          frame True {
            n200 = local read "Green FB Sum"() -> (w393:i16)
            n201 = call "Slower PID.vi"("process variable"=w393, "reset?"="Green FB Reset", "setpoint"="Green FB Setpoint", "PID gains (x 2^8)"="Green FB Gains", "output range"=cluster{"output high":i16, "output low":i16} {"output high"=32767, "output low"=-32768} ("Green FB output range")) -> ("output"=w401:i16)  [unwired: 10 out]
            n202 = To Long Integer(number=w401) -> (32bit integer=w394:i32)
            n203 = Add(x=w394, y=32768) -> (x+y=w396:i32)
            n204 = To Unsigned Word Integer(number=w396) -> (unsigned 16bit integer=w397:u16)
          }
        }
        n205 = Not(x=w383) -> (.not. x?=w380:bool)
        n206 = Select(t=w372, s=w380, f=w371) -> (s? t:f=w385:u32)
        n207 = Subtract(x=w385, y=w355) -> (x-y=w366:u32)
        n208 = Add(x=w366, y=w364) -> (x+y=w362:u32)
        n209 = feedback-in #19(w380) -> ()
        n210 = Boolean To (0,1)(Boolean=w373) -> (0, 1=w379:i16)
        n211 = To Unsigned Word Integer(number=w379) -> (unsigned 16bit integer=w376:u16)
        n212 = Multiply(x=w376, y=w377) -> (x*y=w378:u16)
      }
    }
  }
  n213 = while "APD 1 Counter" {
    tunnel: w2 -> [_]
    stop <- FALSE stop-if-true
    n214 = flat-sequence {
      frame #0 {
        n215 = xnode "FPGA I/O Method Node"("FPGA I/O In"=refnum<k21> "Connector0/DIO0" ("APD 1 DO"), "Timeout"=-1) -> ()  [unwired: 2 out]
      }
      frame #1 {
        n216 = local read "APD1 int gate"() -> (w412:bool)
        n217 = case shown="False" w412 {
          frame False {
          }
          frame True {
            n218 = local read "APD1 out state"() -> (w413:bool)
            n219 = case shown="True" w413 {
              frame False {
                n220 = local read "APD 1 Counts 0"() -> (w415:u32)
                n221 = Increment(x=w415) -> (x+1=→"APD 1 Counts 0":u32)
              }
              frame True {
                n222 = local read "APD 1 Counts 1"() -> (w417:u32)
                n223 = Increment(x=w417) -> (x+1=→"APD 1 Counts 1":u32)
              }
            }
          }
        }
      }
    }
  }
  n224 = while "RF synth board interlacing timing loop" {
    tunnel: w2 -> [_]
    stop <- FALSE stop-if-true
    # "This loop is stalled until the RF FIFO get a value. With this method we gain additional delay time (because  we allow the rest of the main RF loop to procede while this loop waits to send the switch signals - a form of parallelism). This helps to simplify the main RF code. \n\nThe code also allow optimal interlacing while also controlling trap RF phase. \n\nNote: a lot of work has gone into optimizing these methods and it is unclear how they can be made any faster or better than this (many failed tries). Right now there is essentially ~4 ticks (~90 ns ns) of imperfection in the switching from trap 1 to trap 2. ~2 ticks of no RF (phase reset) then ~2 ticks of trap 2 with the wrong amplitude (T1 amplitude). The total ticks is 200, so not a big error.\n\nPhase can be precisely set for each trap. Phase reset and switching, has similar delays as fsk frequency switching. And phase reset and phase offset changes are also not simultaneous. So we can't perfectly line everything up.\n\nIf you start from amp zero though (as for trap 1), the on switch is perfect. Likewise the off is perfect for trap 2. \n\nThe green laser switching is also perfect because of its reduced duty cycle and delays in fsk switching between 80 and 0 MHz."
    n225 = xnode ("FIFO Read")("Timeout"=-1) -> ("Element"=w464:u16, "FIFO Out"=w460:refnum<k21>)  [unwired: 1 in, 1 out]
    n226 = Equal To 0?(x=w464) -> (x = 0?=w461:bool)
    n227 = Not(x=w461) -> (.not. x?=w418:bool)
    n228 = flat-sequence "BD 1 and 2 RF phase and amplitude switching" {
      tunnel: w418 -> [_]
      tunnel: w453 -> [w568]
      tunnel: w452 -> [w567]
      tunnel: w451 -> [w566]
      tunnel: w450 -> [w565]
      tunnel: w449 -> [w564]
      tunnel: w448 -> [w563]
      tunnel: w447 -> [w562]
      tunnel: w446 -> [w561]
      tunnel: w444 -> [w560]
      tunnel: w443 -> [w559]
      tunnel: w442 -> [w558]
      tunnel: w440 -> [w556]
      tunnel: w439 -> [w555]
      tunnel: w438 -> [w554]
      tunnel: w441 -> [w557]
      tunnel: w445 -> [w553]
      tunnel: w437 -> [w592]
      tunnel: w436 -> [w591]
      tunnel: w435 -> [w590]
      tunnel: w434 -> [w589]
      tunnel: w433 -> [w588]
      tunnel: w432 -> [w587]
      tunnel: w431 -> [w586]
      tunnel: w430 -> [w585]
      tunnel: w429 -> [w584]
      tunnel: w427 -> [w583]
      tunnel: w426 -> [w582]
      tunnel: w425 -> [w581]
      tunnel: w424 -> [w580]
      tunnel: w423 -> [w579]
      tunnel: w422 -> [w578]
      tunnel: w428 -> [w577]
      frame #0 {
        # "Delay to align amp/frequency switching depending on the method used.\n\nCan also give enough time to do the parallel amplitude calculations"
        n229 = call "Wait2"("Count(Ticks)"="Amp switch delay") -> ()  [unwired: 1 out]
      }
      frame #1 {
        w548 = TRUE ("Connector1/DIO30")
        # "make phase offset and phase reset active with buffer transfer"
        n230 = xnode "FPGA I/O Node"("Connector1/DIO29"=w548, "Connector1/DIO30"=w548) -> ()  [unwired: 2 in, 2 out]
      }
      frame #2 {
        w549 = FALSE ("Connector1/DIO15")
        # "write phase restart to buffer and reset udclk"
        n231 = xnode "FPGA I/O Node"("Connector1/DIO29"=w549, "Connector1/DIO30"=w549, "Connector1/DIO15"=FALSE ("Connector1/DIO14")) -> ()  [unwired: 3 in, 3 out]
      }
      frame #3 {
        w551 = TRUE ("Connector1/DIO15")
        # "make phase restart active"
        # "reset WR"
        n232 = xnode "FPGA I/O Node"("Connector1/DIO15"=w551, "Connector1/DIO29"=w551, "Connector1/DIO30"=w551) -> ()  [unwired: 3 in, 3 out]
      }
      frame #4 {
        w552 = FALSE ("Connector1/DIO30")
        # "Address"
        # "set amp byte 1, and reset udclk"
        n233 = xnode "FPGA I/O Node"("Connector1/DIO0"=w568, "Connector1/DIO1"=w567, "Connector1/DIO2"=w566, "Connector1/DIO3"=w565, "Connector1/DIO4"=w564, "Connector1/DIO5"=w563, "Connector1/DIO6"=w562, "Connector1/DIO7"=w561, "Connector1/DIO8"=TRUE, "Connector1/DIO9"=FALSE, "Connector1/DIO10"=FALSE, "Connector1/DIO11"=FALSE, "Connector1/DIO12"=FALSE, "Connector1/DIO13"=TRUE, "Connector1/DIO20"=w553, "Connector1/DIO21"=w560, "Connector1/DIO22"=w559, "Connector1/DIO23"=w558, "Connector1/DIO24"=w557, "Connector1/DIO25"=w556, "Connector1/DIO26"=w555, "Connector1/DIO27"=w554, "Connector1/DIO30"=w552, "Connector1/DIO29"=w552) -> ()  [unwired: 24 in, 24 out]
      }
      frame #5 {
        # "write amp byte 1 to buffer"
        n234 = xnode "FPGA I/O Node"("Connector1/DIO15"=FALSE ("Connector1/DIO14")) -> ()  [unwired: 1 in, 1 out]
      }
      frame #6 {
        # "reset WR"
        n235 = xnode "FPGA I/O Node"("Connector1/DIO15"=TRUE) -> ()  [unwired: 1 in, 1 out]
      }
      frame #7 {
        # "Address"
        # "set amp byte 2"
        n236 = xnode "FPGA I/O Node"("Connector1/DIO0"=w592, "Connector1/DIO1"=w591, "Connector1/DIO2"=w590, "Connector1/DIO3"=w589, "Connector1/DIO4"=w588, "Connector1/DIO5"=w587, "Connector1/DIO6"=w586, "Connector1/DIO7"=w585, "Connector1/DIO8"=TRUE, "Connector1/DIO9"=FALSE, "Connector1/DIO10"=FALSE, "Connector1/DIO11"=FALSE, "Connector1/DIO12"=TRUE, "Connector1/DIO13"=FALSE, "Connector1/DIO20"=w584, "Connector1/DIO21"=w577, "Connector1/DIO22"=w583, "Connector1/DIO23"=w582, "Connector1/DIO24"=w581, "Connector1/DIO25"=w580, "Connector1/DIO26"=w579, "Connector1/DIO27"=w578) -> ()  [unwired: 22 in, 22 out]
      }
      frame #8 {
        # "write amp byte 2"
        n237 = xnode "FPGA I/O Node"("Connector1/DIO15"=FALSE ("Connector1/DIO14")) -> ()  [unwired: 1 in, 1 out]
      }
      frame #9 {
        w600 = TRUE ("Connector1/DIO15")
        # "transfer amp bytes 1 and 2 and reset WR"
        n238 = xnode "FPGA I/O Node"("Connector1/DIO29"=w600, "Connector1/DIO30"=w600, "Connector1/DIO15"=TRUE ("Connector1/DIO14")) -> ()  [unwired: 3 in, 3 out]
      }
      frame #10 {
        w602 = FALSE ("Connector1/DIO14")
        # "reset udclk"
        n239 = xnode "FPGA I/O Node"("Connector1/DIO29"=w602, "Connector1/DIO30"=w602) -> ()  [unwired: 2 in, 2 out]
      }
    }
    n240 = flat-sequence "FSK BD 1 (trap X)" {
      tunnel: w418 -> [w466]
      tunnel: [w466] -> w421
      tunnel: w421 -> [w467]
      frame #0 {
        n241 = call "Wait"("Count(Ticks)"="BD 1 Delay (ticks)") -> ()  [unwired: 1 out]
      }
      frame #1 {
        # "switch frequency"
        n242 = xnode "FPGA I/O Node"("Connector1/DIO36"=w467) -> ()  [unwired: 1 in, 1 out]
      }
    }
    n243 = flat-sequence "FSK BD 2 (trap Y or green laser AOM)" {
      tunnel: w418 -> [w604]
      tunnel: [w604] -> w463
      tunnel: w463 -> [w605]
      frame #0 {
        n244 = call "Wait3"("Count(Ticks)"="BD 2 Delay (Ticks)") -> ()  [unwired: 1 out]
      }
      frame #1 {
        # "switch frequency"
        n245 = xnode "FPGA I/O Node"("Connector1/DIO37"=w605) -> ()  [unwired: 1 in, 1 out]
      }
    }
    n246 = xnode ("FIFO Read")("Timeout"=-1, "FIFO In"=w460) -> ("Element"=w455:u16, "FIFO Out"=w459:refnum<k21>)  [unwired: 1 out]
    n247 = xnode ("FIFO Read")("Timeout"=-1, "FIFO In"=w459) -> ("Element"=w454:u16)  [unwired: 2 out]
    n248 = node-c288() -> (w457:T7)  [unwired: 1 in]
    n249 = timed-loop "Convert amplitude words to bits" {
      timing: w457 -> [_]
      timing-out: [_] -> w456
      tunnel: w455 -> [w524]
      tunnel: w454 -> [w523]
      tunnel: [w500] -> w453
      tunnel: [w499] -> w452
      tunnel: [w498] -> w451
      tunnel: [w497] -> w450
      tunnel: [w496] -> w449
      tunnel: [w495] -> w448
      tunnel: [w494] -> w447
      tunnel: [w493] -> w446
      tunnel: [w492] -> w445
      tunnel: [w491] -> w444
      tunnel: [w490] -> w443
      tunnel: [w489] -> w442
      tunnel: [w488] -> w441
      tunnel: [w487] -> w440
      tunnel: [w486] -> w439
      tunnel: [w485] -> w438
      tunnel: [w484] -> w437
      tunnel: [w483] -> w436
      tunnel: [w482] -> w435
      tunnel: [w481] -> w434
      tunnel: [w480] -> w433
      tunnel: [w479] -> w432
      tunnel: [w478] -> w431
      tunnel: [w477] -> w430
      tunnel: [w476] -> w429
      tunnel: [w475] -> w428
      tunnel: [w474] -> w427
      tunnel: [w473] -> w426
      tunnel: [w472] -> w425
      tunnel: [w471] -> w424
      tunnel: [w470] -> w423
      tunnel: [w469] -> w422
      stop <- TRUE stop-if-true
      # "Board 1 Data"
      # "Board 2 Data"
      # "Board 1 Data"
      # "Board 2 Data"
      n250 = Split Number(x=w524) -> (hi(x)=w522:u8, lo(x)=w502:u8)
      n251 = Split Number(x=w523) -> (hi(x)=w521:u8, lo(x)=w501:u8)
      n252 = Number To Boolean Array(number=w522) -> (Boolean array=w542:bool[])
      n253 = Number To Boolean Array(number=w521) -> (Boolean array=w533:bool[])
      n254 = Index Array(array=w542, index=7) -> (element=w500:bool)
      n255 = Index Array(array=w542, index=6) -> (element=w499:bool)
      n256 = Index Array(array=w542, index=5) -> (element=w498:bool)
      n257 = Index Array(array=w542, index=4) -> (element=w497:bool)
      n258 = Index Array(array=w542, index=3) -> (element=w496:bool)
      n259 = Index Array(array=w542, index=2) -> (element=w495:bool)
      n260 = Index Array(array=w542, index=1) -> (element=w494:bool)
      n261 = Index Array(array=w542, index=0) -> (element=w493:bool)
      n262 = Index Array(array=w533, index=7) -> (element=w492:bool)
      n263 = Index Array(array=w533, index=6) -> (element=w491:bool)
      n264 = Index Array(array=w533, index=5) -> (element=w490:bool)
      n265 = Index Array(array=w533, index=4) -> (element=w489:bool)
      n266 = Index Array(array=w533, index=3) -> (element=w488:bool)
      n267 = Index Array(array=w533, index=2) -> (element=w487:bool)
      n268 = Index Array(array=w533, index=1) -> (element=w486:bool)
      n269 = Index Array(array=w533, index=0) -> (element=w485:bool)
      n270 = Number To Boolean Array(number=w502) -> (Boolean array=w520:bool[])
      n271 = Number To Boolean Array(number=w501) -> (Boolean array=w511:bool[])
      n272 = Index Array(array=w520, index=7) -> (element=w484:bool)
      n273 = Index Array(array=w520, index=6) -> (element=w483:bool)
      n274 = Index Array(array=w520, index=5) -> (element=w482:bool)
      n275 = Index Array(array=w520, index=4) -> (element=w481:bool)
      n276 = Index Array(array=w520, index=3) -> (element=w480:bool)
      n277 = Index Array(array=w520, index=2) -> (element=w479:bool)
      n278 = Index Array(array=w520, index=1) -> (element=w478:bool)
      n279 = Index Array(array=w520, index=0) -> (element=w477:bool)
      n280 = Index Array(array=w511, index=7) -> (element=w476:bool)
      n281 = Index Array(array=w511, index=6) -> (element=w475:bool)
      n282 = Index Array(array=w511, index=5) -> (element=w474:bool)
      n283 = Index Array(array=w511, index=4) -> (element=w473:bool)
      n284 = Index Array(array=w511, index=3) -> (element=w472:bool)
      n285 = Index Array(array=w511, index=2) -> (element=w471:bool)
      n286 = Index Array(array=w511, index=1) -> (element=w470:bool)
      n287 = Index Array(array=w511, index=0) -> (element=w469:bool)
    }
    n288 = node-c288(w456) -> ()
  }
  n289 = while "APD 1 Gating" {
    shift-right: [w609] -> _
    shift-left: w2 -> [w614]
    shift-right: [w608] -> _
    shift-left: w4 -> [w606]
    stop <- FALSE stop-if-true
    n290 = flat-sequence {
      tunnel: w614 -> [w617]
      tunnel: [w618] -> w612
      tunnel: [w617] -> w610
      tunnel: [w616] -> w607
      tunnel: w606 -> [w616]
      tunnel: [w621] -> w613
      tunnel: w612 -> [w621]
      tunnel: [w620] -> w611
      tunnel: w610 -> [w620]
      tunnel: w607 -> [w619]
      tunnel: [w639] -> w609
      tunnel: w613 -> [w653]
      tunnel: w611 -> [w650]
      tunnel: [w622] -> w608
      frame #0 {
        n291 = call "Loop Timer4"("Count(Ticks)"=w617) -> ("Tick Count(Ticks)"=w618:u32)
      }
      frame #1 {
        # "Signal maybe then sent through \na transistor before APD"
        n292 = xnode "FPGA I/O Node"("Connector1/DIO33"=w619) -> ()  [unwired: 1 in, 1 out]
        "APD1 int gate" <- w619
      }
      frame #2 {
        n293 = feedback #20(TRUE) -> (w645:bool)
        n294 = feedback-in #21(w653) -> ()
        n295 = feedback #21(w653) -> (w652:u32)
        n296 = Not(x=w645) -> (.not. x?=w642:bool)
        n297 = feedback-in #20(w642) -> ()
        n298 = Subtract(x=w653, y=w652) -> (x-y=w651:u32)
        n299 = Select(t="APD Gate ON Count", s=w642, f="APD Gate OFF Count") -> (s? t:f=w647:u16)
        n300 = Subtract(x=w651, y=w650) -> (x-y=w627:u32)
        n301 = Subtract(x=w647, y=w627) -> (x-y=w638:u32)
        n302 = Number To Boolean Array(number=w627) -> (Boolean array=w628:bool[])
        n303 = Or Array Elements(Boolean array=w628) -> (logical OR=w626:bool)
        n304 = Boolean To (0,1)(Boolean="+ phase (APD 1 Gate)") -> (0, 1=w636:i16)
        n305 = Boolean To (0,1)(Boolean=w626) -> (0, 1=w633:i16)
        n306 = Multiply(x=w636, y="Phase count adjustment (APD 1 Gate)") -> (x*y=w634:i16)
        n307 = To Unsigned Byte Integer(number=w633) -> (unsigned 8bit integer=w630:u8)
        n308 = Add(x=w638, y=w634) -> (x+y=w639:u32)
        n309 = feedback #22(i16 0) -> (w641:i16)
        n310 = Subtract(x=w641, y=w634) -> (x-y=w640:i16)
        "APD 1 Gate Relative Phase" <- w640
        n311 = feedback-in #22(w640) -> ()
        n312 = feedback #23(u8 0) -> (w631:u8)
        n313 = Add(x=w630, y=w631) -> (x+y=w629:u8)
        "APD 1 Gate Late Counter" <- w629
        n314 = feedback-in #23(w629) -> ()
        n315 = case shown="2" "APD Gate Operating Mode" {
          tunnel: [TRUE FALSE w656] -> w623
          tunnel: w645 -> [_ _ w656]
          frame 0, Default {
          }
          frame 1 {
          }
          frame 2 {
          }
        }
        n316 = Not(x=w623) -> (.not. x?=w624:bool)
        n317 = Select(t=w624, s="Invert APD Gate", f=w623) -> (s? t:f=w622:bool)
      }
    }
  }
  n318 = while "APD 2 Gating" {
    shift-right: [w660] -> _
    shift-left: w2 -> [w665]
    shift-right: [w659] -> _
    shift-left: w4 -> [w657]
    stop <- FALSE stop-if-true
    n319 = flat-sequence {
      tunnel: w665 -> [w668]
      tunnel: [w669] -> w663
      tunnel: [w668] -> w661
      tunnel: [w667] -> w658
      tunnel: w657 -> [w667]
      tunnel: [w672] -> w664
      tunnel: w663 -> [w672]
      tunnel: [w671] -> w662
      tunnel: w661 -> [w671]
      tunnel: w658 -> [w670]
      tunnel: [w694] -> w660
      tunnel: w664 -> [w704]
      tunnel: w662 -> [w702]
      tunnel: [w673] -> w659
      frame #0 {
        n320 = call "Loop Timer3"("Count(Ticks)"=w668) -> ("Tick Count(Ticks)"=w669:u32)
      }
      frame #1 {
        # "Signal maybe then sent through \na transistor before APD"
        n321 = xnode "FPGA I/O Node"("Connector1/DIO34"=w670) -> ()  [unwired: 1 in, 1 out]
        "APD2 int gate" <- w670
      }
      frame #2 {
        n322 = local read "APD Gate ON Count"() -> (w687:u16)
        n323 = local read "APD Gate OFF Count"() -> (w686:u16)
        n324 = feedback #24(TRUE) -> (w699:bool)
        n325 = feedback-in #25(w704) -> ()
        n326 = feedback #25(w704) -> (w688:u32)
        n327 = Not(x=w699) -> (.not. x?=w697:bool)
        n328 = feedback-in #24(w697) -> ()
        n329 = Subtract(x=w704, y=w688) -> (x-y=w703:u32)
        n330 = Select(t=w687, s=w697, f=w686) -> (s? t:f=w701:u16)
        n331 = Subtract(x=w703, y=w702) -> (x-y=w679:u32)
        n332 = Subtract(x=w701, y=w679) -> (x-y=w693:u32)
        n333 = Number To Boolean Array(number=w679) -> (Boolean array=w678:bool[])
        n334 = Or Array Elements(Boolean array=w678) -> (logical OR=w677:bool)
        n335 = Boolean To (0,1)(Boolean="+ phase (APD 2 Gate)") -> (0, 1=w691:i16)
        n336 = Multiply(x=w691, y="Phase count adjustment (APD 2 Gate)") -> (x*y=w689:i16)
        n337 = Boolean To (0,1)(Boolean=w677) -> (0, 1=w684:i16)
        n338 = Add(x=w693, y=w689) -> (x+y=w694:u32)
        n339 = To Unsigned Byte Integer(number=w684) -> (unsigned 8bit integer=w681:u8)
        n340 = feedback #26(i16 0) -> (w696:i16)
        n341 = Subtract(x=w696, y=w689) -> (x-y=w695:i16)
        "APD 2 Gate Relative Phase" <- w695
        n342 = feedback-in #26(w695) -> ()
        n343 = feedback #27(u8 0) -> (w682:u8)
        n344 = Add(x=w681, y=w682) -> (x+y=w680:u8)
        "APD 2 Gate Late Counter" <- w680
        n345 = feedback-in #27(w680) -> ()
        n346 = local read "APD Gate Operating Mode"() -> (w685:u8)
        n347 = case shown="2" w685 {
          tunnel: [TRUE FALSE w707] -> w674
          tunnel: w699 -> [_ _ w707]
          frame 0, Default {
          }
          frame 1 {
          }
          frame 2 {
          }
        }
        n348 = local read "Invert APD Gate"() -> (w676:bool)
        n349 = Not(x=w674) -> (.not. x?=w675:bool)
        n350 = Select(t=w675, s=w676, f=w674) -> (s? t:f=w673:bool)
      }
    }
  }
  n351 = while "Trap RF control, main calculations (raster scanning, intensity and position feedback, phase control etc) with primary timing trigger" {
    shift-right: [w722] -> _
    shift-left: w2 -> [w721]
    shift-right: [w720] -> _
    shift-left: FALSE ("Swap F1 and F2") -> [w719]
    shift-right: [w715] -> _
    shift-left: u16 0 ("BD 1 Amplitude 3") -> [w712]
    shift-right: [w714] -> _
    shift-left: u16 0 ("BD 2 Amplitude 3") -> [w710]
    shift-right: [w709] -> _
    shift-left: u64 0 -> [w708]
    stop <- FALSE stop-if-true
    n352 = flat-sequence {
      tunnel: w719 -> [w728]
      tunnel: w721 -> [w725]
      tunnel: [w728] -> w718
      tunnel: [w724] -> w717
      tunnel: [w725] -> w716
      tunnel: [w727] -> w713
      tunnel: w712 -> [w727]
      tunnel: [w726] -> w711
      tunnel: w710 -> [w726]
      tunnel: [w739] -> w722
      tunnel: [w738] -> w720
      tunnel: w718 -> [w737]
      tunnel: w717 -> [w736]
      tunnel: w716 -> [w735]
      tunnel: [w734] -> w715
      tunnel: [w733] -> w714
      tunnel: w713 -> [w732]
      tunnel: w711 -> [w731]
      tunnel: [w730] -> w709
      tunnel: w708 -> [w729]
      frame #0 {
        n353 = call "Loop Timer2"("Count(Ticks)"=w725) -> ("Tick Count(Ticks)"=w724:u32)
      }
      frame #1 {
        n354 = flat-sequence {
          tunnel: w737 -> [w747]
          tunnel: w732 -> [w741]
          tunnel: w731 -> [w740]
          tunnel: [w807] -> w739
          tunnel: [w819] -> w738
          tunnel: w736 -> [w813]
          tunnel: w735 -> [w810]
          tunnel: [w758] -> w734
          tunnel: [w757] -> w733
          tunnel: [w749] -> w730
          tunnel: w729 -> [w748]
          frame #0 {
            w742 = -1 ("Timeout")
            # "Operation when you need a long delay for either X or Y to synchonize AOD light out phase (> ~100 ticks)\nor want shorter trap ON timing. Puts some of the delay timing in parallel with the later computations."
            # "Trigger the external loop by sending the boolean FSK value through a FIFO.\nTiming is precise."
            n355 = Boolean To (0,1)(Boolean=w747) -> (0, 1=w746:i16)
            n356 = To Unsigned Word Integer(number=w746) -> (unsigned 16bit integer=w745:u16)
            n357 = xnode ("FIFO Method Node")("Element"=w745, "Timeout"=w742) -> ("FIFO Out"=w744:refnum<k21>)  [unwired: 1 in, 1 out]
            n358 = xnode ("FIFO Method Node")("Element"=w741, "Timeout"=w742, "FIFO In"=w744) -> ("FIFO Out"=w743:refnum<k21>)  [unwired: 1 out]
            n359 = xnode ("FIFO Method Node")("Element"=w740, "Timeout"=w742, "FIFO In"=w743) -> ()  [unwired: 2 out]
          }
          frame #1 {
            # "Just counts, wraps around, 8 bit"
            # "Which trap cycle"
            # "Only save the 3rd set's amp in the loop"
            # "If this is NOT set 3 AND NOT (RF synth controls green AND green FB running)\nthen use this sets amp value (otherwise keep the green feedback value)"
            # "Just flips back and forth."
            # "If interlacing is off, this is which cycle to use."
            # "Keep track of trap cycles (trap 1, 2, 3...)"
            # "This is the prior cycle's on time"
            # "increment timing\nindex, reset to 0 if \nend of matrix"
            # "Reset to begginning (1) when number of cycles reached."
            # "timing index"
            # "build byte stacks for writing data\n(must correspond to addresses array constant)"
            # "Timing housekeeping"
            # "Adjust phase if late\n(maintains constant phase relationship between cycles)"
            n360 = feedback #28(u8 0 ("t")) -> (w816:u8)
            n361 = Increment(x=w816) -> (x+1=w855:u8)
            n362 = Increment(x="Number Interlace Cycles") -> (x+1=w850:u8)
            n363 = Equal?(x=w855, y=w850) -> (x = y?=w857:bool)
            n364 = Select(t=u8 1, s=w857, f=w855) -> (s? t:f=w815:u8)
            n365 = feedback-in #28(w815) -> ()
            n366 = Increment(x=w815) -> (x+1=w852:u8)
            n367 = Equal?(x=w852, y=w850) -> (x = y?=w853:bool)
            n368 = Select "This cycle"(t=u8 1, s=w853, f=w852) -> (s? t:f=w849:u8)
            n369 = Select(t=w849, s="Interlace ON/OFF", f="Interlace Off Parameters") -> (s? t:f=w768:u8)
            n370 = feedback-in #29(w813) -> ()
            n371 = feedback #29(w813) -> (w812:u32)
            n372 = Select(t=w815, s="Interlace ON/OFF", f="Interlace Off Parameters") -> (s? t:f=w848:u8)
            n373 = Subtract(x=w813, y=w812) -> (x-y=w811:u32)
            n374 = Subtract "The error"(x=w811, y=w810) -> (x-y=w794:u32)
            n375 = case shown="1, Default" w848 {
              tunnel: ["DIO count 1 (ticks)" "DIO count 2 (ticks)" "DIO count 3 (ticks)"] -> w809
              frame 1, Default {
              }
              frame 2 {
              }
              frame 3 {
              }
            }
            n376 = Number To Boolean Array(number=w794) -> (Boolean array=w795:bool[])
            n377 = Or Array Elements(Boolean array=w795) -> (logical OR=w793:bool)
            n378 = Boolean To (0,1)(Boolean=w793) -> (0, 1=w800:i16)
            n379 = To Unsigned Byte Integer(number=w800) -> (unsigned 8bit integer=w797:u8)
            n380 = feedback #30(u8 0) -> (w798:u8)
            n381 = Add(x=w797, y=w798) -> (x+y=w796:u8)
            "DIO Late Counter" <- w796
            n382 = feedback-in #30(w796) -> ()
            n383 = Subtract(x=w809, y=w794) -> (x-y=w808:u32)
            n384 = disable-structure shown="Disabled" {
              disable-tunnel: [w861 _] -> w792
              disable-tunnel: w768 -> [w858 _]
              frame Disabled {
                n385 = feedback #31(i64 0 ("y")) -> (w860:i64)
                n386 = case "Synchronize trap oscillations - always begin/end with trap 1" shown="1, Default" w858 {
                  tunnel: [w862 w863 w864] -> w861
                  tunnel: w860 -> [w862 w863 _]
                  frame 2 {
                  }
                  frame 3 {
                  }
                  frame 1, Default {
                    n387 = Or(x="Osc traps", y="Initiate trap osc") -> (x .or. y?=w866:bool)
                    n388 = case "Trap sine oscillation (or whatever pattern is stored in memory)" shown="True" w866 {
                      tunnel: [i64 0 ("y") w870] -> w864
                      tunnel: "Initiate trap osc" -> [_ w873]
                      frame False {
                      }
                      frame True {
                        w877 = u16 0
                        w875 = -1
                        n389 = local write "Initiate trap osc"(FALSE ("Initiate trap osc")) -> ()
                        n390 = feedback #32(w877) -> (w879:u16)
                        n391 = Select(t=w877, s=w873, f=w879) -> (s? t:f=w878:u16)
                        n392 = Greater Or Equal?(x=w878, y="Trap osc period (pts)") -> (x >= y?=w884:bool)
                        n393 = Or(x=w873, y=w884) -> (x .or. y?=w885:bool)
                        n394 = Select(t=u16 0, s=w885, f=w878) -> (s? t:f=w869:u16)
                        n395 = feedback #33(w875) -> (w876:i32)
                        n396 = Select(t=w875, s=w873, f=w876) -> (s? t:f=w874:i32)
                        n397 = Increment(x=w874) -> (x+1=w881:i32)
                        n398 = Equal?(x=w869, y=u16 0) -> (x = y?=w882:bool)
                        n399 = Increment(x=w869) -> (x+1=w889:u16)
                        n400 = feedback-in #32(w889) -> ()
                        n401 = Select(t=w881, s=w882, f=w874) -> (s? t:f=w880:i32)
                        n402 = feedback-in #33(w880) -> ()
                        n403 = case shown="False" "Osc trap cont." {
                          tunnel: w880 -> [w893 _]
                          frame False {
                            n404 = Greater Or Equal?(x=w893, y="N trap osc periods") -> (x >= y?=w891:bool)
                            n405 = Not(x=w891) -> (.not. x?=w890:bool)
                            n406 = local write "Osc traps"(w890) -> ()
                          }
                          frame True {
                          }
                        }
                        n407 = xnode ("Memory Read")("Address"=w869, "Memory In"=refnum<k21> "Trap osc memory") -> ("Data"=w870:i64)  [unwired: 1 out]
                      }
                    }
                  }
                }
                n408 = feedback-in #31(w861) -> ()
              }
              frame Enabled {
              }
            }
            n409 = local read "green FB running"() -> (w781:bool)
            n410 = And(x=w781, y="RF synth bd controls green") -> (x .and. y?=w780:bool)
            n411 = case shown="1, Default" w768 {
              tunnel: [w1020 w1256 "BD 1 Frequency 3"] -> w845
              tunnel: [w1061 w1255 w1277] -> w784
              tunnel: ["BD 2 Amplitude 1" "BD 2 Amplitude 2" w1276] -> w776
              tunnel: [w1017 w1252 "BD 1 Amplitude 3"] -> w758
              tunnel: "FB Gains" -> [w1038 w1262 _]
              tunnel: "FB output range" -> [w1039 w1261 _]
              tunnel: w792 -> [w1036 w1259 _]
              tunnel: "BD 2 Frequency 1" -> [w1033 _ _]
              tunnel: "BD 2 Frequency 2" -> [_ w1255 _]
              tunnel: "BD 2 Frequency 3" -> [_ _ w1277]
              tunnel: w780 -> [_ _ w1275]
              tunnel: [w1020 w1253 w1274] -> w749
              tunnel: w748 -> [w1019 w1253 w1274]
              frame 1, Default {
                w1052 = fxp<+/-,24,9> 0.0 ("AI1 X Set 2")
                w1046 = u16 0
                w1059 = u64 0 ("f")
                # "Changed by Ronen - correction \nby PID is now implemented not on \nthe Base BD1 frequency but on the last\nfrequency sent."
                # "Added by Ronen -\nUpper and Lower \nLimits for the FB \ngenerated frequency\nto avoid losing bead \nwhen tether breaks"
                # "Explanation of raster scanning:\n1. Cycles: increment counter by 1 every time interlace cycle returns to trap 1. As long as \n  Cycle per Step is larger than counter, keep incrementing counter and do not change step counter.\n  Once counter is equal to Cycles per step, zero counter and increment step counter.\n2. Steps: Increments up every time cycles counter equals cycles per step. Performs the following:\n- To determine DIRECTION of frequency change:  If ScanstepX2 is EQUAL to step counter (full for-back scan finished)\n   frequency increment is set to zero, AND step counter is set to zero. \n   Otherwise: if no change to step counter (because cycleperstep>cycle counter), then no change to frequency\n   increment. \n   If step counter has changed (cycleperstep=cycle counter), then need to figure out direction of frequency change:\n   if step counter is EQUAL to Scansteps: No change to frequency increment\n   Otherwise: If scan steps > step counter - 1 (forward scan NOT completed): increment frequency by 1\n                       If scan steps equal or smaller than step counter -1 (forward scan completed): increment frequency by -1\n\n3. Scans: Increment scan counter every time step counter equals 2Xscan steps (full for-back scan completed)\n    if number of scans > scan counter: Send TRUE to scanning, continue scan\n    if number of scans = scan counter: Send FALSE to Scanning, Scan finished.\n\n  The wire with the asterik can be used as the index for getting the mirror positions in the offset scan."
                # "This signal integration happens no matter what\nso that correct setpoints can be chosen before \nturning on the FB."
                # "Trap 1"
                n412 = local read "AI1 X Set 2"() -> (w1031:fxp<+/-,16,1>)
                n413 = local read "AI1 X Set 1"() -> (w1049:fxp<+/-,16,1>)
                n414 = local read "Scanning"() -> (w1062:bool)
                n415 = Multiply(x=w1031, y="B factor") -> (x*y=w1029:fxp<+/-,48,17>)
                n416 = Or(x=w1062, y="Start scan") -> (x .or. y?=w1014:bool)
                n417 = case shown="True" "Diff FB Measurement?" {
                  tunnel: w1029 -> [w1152 w1161]
                  tunnel: w1049 -> [w1151 w1162]
                  tunnel: [w1149 w1153] -> w1050
                  frame False {
                    n418 = Select(t=w1151, s="Trap Pos FB Monitor T1 or T2", f=w1152) -> (s? t:f=w1149:fxp<+/-,48,17>)
                  }
                  frame True {
                    n419 = Subtract(x=w1162, y=w1161) -> (x-y=w1154:fxp<+/-,48,17>)
                    n420 = Not(x="Negate Diff?") -> (.not. x?=w1160:bool)
                    n421 = Boolean To (0,1)(Boolean="Negate Diff?") -> (0, 1=w1158:i16)
                    n422 = Boolean To (0,1)(Boolean=w1160) -> (0, 1=w1159:i16)
                    n423 = Negate(x=w1158) -> (-x=w1157:i16)
                    n424 = Add(x=w1157, y=w1159) -> (x+y=w1155:i16)
                    n425 = Multiply(x=w1155, y=w1154) -> (x*y=w1153:fxp<+/-,63,32>)
                  }
                }
                n426 = feedback #34(w1046) -> (w1045:u16)
                n427 = Increment(x=w1045) -> (x+1=w1047:u16)
                n428 = Greater Or Equal?(x=w1047, y="Trap Pos FB Int Count") -> (x >= y?=w1018:bool)
                n429 = Select(t=w1046, s=w1018, f=w1047) -> (s? t:f=w1048:u16)
                n430 = feedback-in #34(w1048) -> ()
                n431 = feedback #35(w1052) -> (w1051:fxp<+/-,24,9>)
                n432 = Add(x=w1050, y=w1051) -> (x+y=w1044:fxp<+/-,24,9>)
                n433 = Select(t=w1052, s=w1018, f=w1044) -> (s? t:f=w1055:fxp<+/-,24,9>)
                n434 = feedback-in #35(w1055) -> ()
                n435 = case "Trap 1 X intensity feedback" shown="True" "FB On/Off Set 1" {
                  tunnel: "BD 1 Amplitude 1" -> [w1244 _]
                  tunnel: [w1244 w1248] -> w1017
                  tunnel: w1039 -> [_ w1245]
                  tunnel: w1038 -> [_ w1246]
                  frame False {
                  }
                  frame True {
                    n436 = local read "AI2 Y Sum Set 1"() -> (w1249:i16)
                    n437 = call "Slower PID.vi"("process variable"=w1249, "reset?"="FB Reset Set 1", "setpoint"="FB Setpoint Set 1", "PID gains (x 2^8)"=w1246, "output range"=w1245) -> ("output"=w1250:i16)  [unwired: 10 out]
                    n438 = To Unsigned Word Integer(number=w1250) -> (unsigned 16bit integer=w1248:u16)
                  }
                }
                "BD1 amplitude 1 out" <- w1017
                n439 = Divide(x=w1044, y="Trap Pos FB Int Count") -> (x/y=w1015:fxp<+/-,16,1>)
                n440 = case "For raster scanning" shown="True" w1014 {
                  tunnel: [u64 0 w1092] -> w1016
                  tunnel: [FALSE w1080] -> w1009
                  tunnel: [i16 0 w1079] -> w1010
                  tunnel: w1015 -> [_ w1078]
                  tunnel: "Start scan" -> [_ w1072]
                  frame False {
                    n441 = local write "Scanning"(FALSE ("scanning")) -> ()
                  }
                  frame True {
                    w1086 = u64 0
                    # "Changed by RG, to introduce force\ndependent stopping of the raster scan \nand manual stopping"
                    # "count number of cycles"
                    n442 = feedback #36(w1086) -> (w1089:u64)
                    n443 = Select(t=w1086, s=w1072, f=w1089) -> (s? t:f=w1091:u64)
                    n444 = Increment(x=w1091) -> (x+1=w1084:u64)
                    n445 = Equal?(x=i16 1, y=w1084) -> (x = y?=w1082:bool)
                    n446 = And(x="Abort scan", y=w1082) -> (x .and. y?=w1080:bool)
                    n447 = Greater?(x="Cycles per step", y=w1084) -> (0:w1087:bool)
                    n448 = Select(t=w1084, s=w1087, f=w1086) -> (s? t:f=w1088:u64)
                    n449 = feedback-in #36(w1088) -> ()
                    n450 = Greater?(x=w1078, y="Raster setpoint") -> (0:w1075:bool)
                    n451 = And(x=w1075, y="Raster to target force") -> (x .and. y?=w1073:bool)
                    n452 = case shown="False" w1080 {
                      tunnel: [w1099 i16 0] -> w1092
                      tunnel: w1072 -> [w1124 _]
                      tunnel: w1087 -> [w1117 _]
                      tunnel: w1086 -> [w1107 _]
                      tunnel: [w1101 FALSE] -> w1081
                      tunnel: [w1097 w1135] -> w1079
                      tunnel: [w1100 w1136] -> w1076
                      frame False {
                        w1108 = i64 0
                        # "scan incr."
                        # "freq. incr. mult."
                        # "count steps"
                        n453 = feedback #37(w1107) -> (w1132:u64)
                        n454 = Select(t=w1107, s=w1124, f=w1132) -> (s? t:f=w1100:u64)
                        n455 = Increment(x=w1100) -> (x+1=w1131:u64)
                        n456 = Add(x="Scan steps", y="Scan steps") -> (x+y=w1130:u64)
                        n457 = Select(t=w1100, s=w1117, f=w1131) -> (s? t:f=w1112:u64)
                        n458 = Greater?(x=w1130, y=w1112) -> (0:w1111:bool)
                        n459 = Select(t=w1112, s=w1111, f=w1107) -> (s? t:f=w1128:u64)
                        n460 = feedback-in #37(w1128) -> ()
                        n461 = Equal?(x="Scan steps", y=w1112) -> (x = y?=w1116:bool)
                        n462 = Greater?(x="Scan steps", y=w1100) -> (0:w1127:bool)
                        n463 = feedback #38(w1108) -> (w1129:i64)
                        n464 = Select(t=w1108, s=w1124, f=w1129) -> (s? t:f=w1114:i64)
                        n465 = Increment(x=w1114) -> (x+1=w1126:i64)
                        n466 = Decrement(x=w1114) -> (x-1=w1125:i64)
                        n467 = Select(t=w1126, s=w1127, f=w1125) -> (s? t:f=w1115:i64)
                        n468 = Select(t=w1114, s=w1116, f=w1115) -> (s? t:f=w1113:i64)
                        n469 = Select(t=w1114, s=w1117, f=w1113) -> (s? t:f=w1109:i64)
                        n470 = Select(t=w1109, s=w1111, f=w1108) -> (s? t:f=w1110:i64)
                        n471 = feedback-in #38(w1110) -> ()
                        n472 = feedback #39(w1107) -> (w1123:u64)
                        n473 = Select(t=w1107, s=w1124, f=w1123) -> (s? t:f=w1119:u64)
                        n474 = Increment(x=w1119) -> (x+1=w1120:u64)
                        n475 = Select(t=w1119, s=w1111, f=w1120) -> (s? t:f=w1118:u64)
                        n476 = Greater?(x="Number of scans", y=w1118) -> (0:w1104:bool)
                        n477 = Multiply(x="Scan freq.  increment", y=w1114) -> (x*y=w1099:i64)
                        n478 = Select(t=TRUE, s="Cont. Scan", f=w1104) -> (s? t:f=w1101:bool)
                        n479 = Select(t=w1118, s=w1101, f=w1107) -> (s? t:f=w1121:u64)
                        n480 = feedback-in #39(w1121) -> ()
                        n481 = local read "BD 1 Frequency 1"() -> (w1098:u64)
                        n482 = Increment(x=w1118) -> (x+1=→"Scan I":u64)
                        n483 = Add(x=w1099, y=w1098) -> (x+y=w1097:u64)
                        "Actual Scan freq" <- w1097
                      }
                      frame True {
                        n484 = local read "Actual Scan freq"() -> (w1135:u64)
                        n485 = local read "Scan steps"() -> (w1136:u64)
                      }
                    }
                    "Scanning" <- w1081
                    n486 = case shown="True" w1073 {
                      tunnel: w1076 -> [_ w1096]
                      frame False {
                      }
                      frame True {
                        n487 = Add(x=w1096, y=i16 2) -> (x+y=w1094:u64)
                        n488 = local write "Raster to target force"(FALSE) -> ()
                        n489 = local write "Scan steps"(w1094) -> ()
                      }
                    }
                  }
                }
                n490 = feedback #40(fxp<+/-,24,9> 0.0 ("AI1 X Set 2")) -> (w1056:fxp<+/-,24,9>)
                n491 = Select(t=w1044, s=w1018, f=w1056) -> (s? t:f=w1057:fxp<+/-,24,9>)
                "Trap Pos FB Int Signal" <- w1057
                n492 = feedback-in #40(w1057) -> ()
                n493 = feedback #41(fxp<+/-,16,1> 0.0 ("Trap Pos FB Int-Norm Signal")) -> (w1041:fxp<+/-,16,1>)
                n494 = Select(t=w1015, s=w1018, f=w1041) -> (s? t:f=w1040:fxp<+/-,16,1>)
                "Trap Pos FB Int-Norm Signal" <- w1040
                n495 = feedback-in #41(w1040) -> ()
                n496 = case "For position feedback" shown="True" "Force feedback" {
                  tunnel: [i64 0 w1168] -> w1025
                  tunnel: w1015 -> [_ w1165]
                  tunnel: w1018 -> [_ w1164]
                  frame False {
                  }
                  frame True {
                    n497 = feedback #42(i64 0) -> (w1167:i64)
                    n498 = case shown="True" w1164 {
                      tunnel: [w1169 w1173] -> w1168
                      tunnel: w1167 -> [w1169 _]
                      tunnel: w1165 -> [_ w1172]
                      frame False {
                      }
                      frame True {
                        n499 = xnode ("PID")("process variable"=w1172, "reset?"="Trap Pos. FB Reset", "setpoint"="Trap Pos. FB SP", "PID gains"="Trap Pos. FB Gains", "output range"="Trap pos. FB Range") -> ("output"=w1182:fxp<+/-,16,1>)
                        n500 = Negate(x=w1182) -> (-x=w1181:fxp<+/-,17,2>)
                        n501 = Select(t=w1181, s="Trap Pos FB Negate Action", f=w1182) -> (s? t:f=w1178:fxp<+/-,17,2>)
                        n502 = Scale By Power Of 2(n=u32 15, x=u32 1) -> (x*2^n=w1175:u32)
                        n503 = Multiply(x=w1178, y=w1175) -> (x*y=w1174:fxp<+/-,17,17>)
                        n504 = To Quad Integer(1:w1174) -> (0:w1186:i64)
                        "Trap Pos FB Action" <- w1186
                        n505 = Multiply(x=w1186, y="Trap Pos. FB Mult Factor") -> (x*y=w1184:i64)
                        n506 = Add(x=w1184, y="Trap Pos. FB Offset Factor") -> (x+y=w1173:i64)
                        n507 = disable-structure shown="Disabled" {
                          disable-tunnel: w1173 -> [w1193 _]
                          frame Disabled {
                            w1197 = u32 0
                            n508 = feedback #43() -> (w1194:i64)  [unwired: 1 in]
                            n509 = Add(x=w1193, y=w1194) -> (x+y=w1191:i64)
                            n510 = feedback #44(w1197) -> (w1199:u32)
                            n511 = Increment(x=w1199) -> (x+1=w1188:u32)
                            n512 = Greater Or Equal?(x=w1188, y="FB Trig Integrate") -> (x >= y?=w1189:bool)
                            n513 = Select(t=i64 0, s=w1189, f=w1191) -> (s? t:f=w1195:i64)
                            n514 = feedback-in #43(w1195) -> ()
                            n515 = Select(t=w1197, s=w1189, f=w1188) -> (s? t:f=w1198:u32)
                            n516 = feedback-in #44(w1198) -> ()
                            n517 = And(x=w1189, y="FPGA Trap Trig") -> (x .and. y?=w1196:bool)
                            n518 = case "Trap FB trigger excitation laser ON" shown="True" w1196 {
                              tunnel: w1191 -> [_ w1203]
                              tunnel: w1188 -> [_ w1201]
                              frame False {
                              }
                              frame True {
                                n519 = Not(x="TTrig Negate Pos") -> (.not. x?=w1210:bool)
                                n520 = Boolean To (0,1)(Boolean="TTrig Negate Pos") -> (0, 1=w1208:i16)
                                n521 = Boolean To (0,1)(Boolean=w1210) -> (0, 1=w1209:i16)
                                n522 = Negate(x=w1208) -> (-x=w1207:i16)
                                n523 = Add(x=w1207, y=w1209) -> (x+y=w1206:i16)
                                n524 = Multiply(x=w1206, y=w1203) -> (x*y=w1205:i64)
                                "TTrig Sig" <- w1205
                                n525 = Multiply(x="FPGA TTrig Thresh", y=w1201) -> (x*y=w1202:i64)
                                "TTrig Fin Thresh" <- w1202
                                n526 = Greater Or Equal?(x=w1205, y=w1202) -> (x >= y?=w1204:bool)
                                n527 = case shown="True" w1204 {
                                frame False {
                                }
                                frame True {
                                w1213 = TRUE ("Green FB On/Off")
                                w1215 = u8 2 ("Operating Mode")
                                n528 = local write "Operating Mode"(w1215) -> ()
                                n529 = local write item#-1(w1215) -> ()
                                n530 = local write item#-1(w1213) -> ()
                                n531 = local write "FPGA Trap Trig"(FALSE ("FPGA Trap Trig")) -> ()
                                "TTrig?" <- w1213
                                }
                                }
                              }
                            }
                          }
                          frame Enabled {
                          }
                        }
                      }
                    }
                    n532 = feedback-in #42(w1168) -> ()
                  }
                }
                n533 = And(x="Force feedback", y="Dynamic Force FB (Ronen)") -> (x .and. y?=w1026:bool)
                n534 = case shown="True" w1026 {
                  tunnel: w1025 -> [w1140 w1144]
                  tunnel: [w1139 w1143] -> w1011
                  tunnel: w1019 -> [_ w1142]
                  tunnel: w1018 -> [_ w1141]
                  frame False {
                    # "(BD1 Frequency 1)"
                    n535 = Add(x="BD 1 Frequency 1", y=w1140) -> (x+y=w1139:u64)
                  }
                  frame True {
                    n536 = case shown="True" w1141 {
                      tunnel: w1144 -> [_ w1148]
                      tunnel: [w1145 w1147] -> w1143
                      tunnel: w1142 -> [w1145 w1146]
                      frame False {
                      }
                      frame True {
                        n537 = Add(x=w1146, y=w1148) -> (x+y=w1147:u64)
                      }
                    }
                  }
                }
                n538 = case shown="True" w1009 {
                  tunnel: [w1065 w1067] -> w1012
                  tunnel: w1011 -> [w1065 _]
                  tunnel: w1010 -> [_ w1067]
                  frame False {
                  }
                  frame True {
                    n539 = local write "BD 1 Frequency 1"(w1067) -> ()
                    n540 = local write "Abort scan"(FALSE) -> ()
                  }
                }
                n541 = Select(t=w1036, s="Trap 1 osc enable", f=i64 0) -> (s? t:f=w1034:i64)
                n542 = Select(t=w1059, s="Scan BD", f=w1016) -> (s? t:f=w1058:u64)
                n543 = Select(t=w1016, s="Scan BD", f=w1059) -> (s? t:f=w1024:u64)
                n544 = Add(x=w1058, y=w1033) -> (x+y=w1061:u64)
                n545 = Compound Arithmetic op=ADD(w1034, w1012, w1024) -> (w1023:u64)
                n546 = In Range and Coerce(upper limit="FB Max Frequency", x=w1023, lower limit="FB Min frequency") -> (coerced(x)=w1020:u64)  [unwired: 1 out]
                "BD1 Frequency Out 1" <- w1020
              }
              frame 2 {
                # "Trap 2"
                n547 = case "Trap 2 X intensity feedback" shown="True" "FB On/Off Set 2" {
                  tunnel: [w1266 w1269] -> w1252
                  tunnel: "BD 1 Amplitude 2" -> [w1266 _]
                  tunnel: w1262 -> [_ w1268]
                  tunnel: w1261 -> [_ w1267]
                  frame False {
                  }
                  frame True {
                    n548 = local read "AI2 Y Sum Set 2"() -> (w1272:i16)
                    n549 = call "Slower PID.vi"("process variable"=w1272, "reset?"="FB Reset Set 2", "setpoint"="FB Setpoint Set 2", "PID gains (x 2^8)"=w1268, "output range"=w1267) -> ("output"=w1270:i16)  [unwired: 10 out]
                    n550 = To Unsigned Word Integer(number=w1270) -> (unsigned 16bit integer=w1269:u16)
                  }
                }
                "BD1 amplitude 2 out" <- w1252
                n551 = Select(t=w1259, s="Trap 2 osc enable", f=i64 0) -> (s? t:f=w1258:i64)
                n552 = Add(x="BD 1 Frequency 2", y=w1258) -> (x+y=w1256:u64)
                "BD1 Frequency Out 2" <- w1256
              }
              frame 3 {
                # "Fluorescence period"
                n553 = disable-structure shown="Disabled" {
                  disable-tunnel: [w1285 _] -> w1276
                  disable-tunnel: w1275 -> [w1284 _]
                  frame Disabled {
                    # "Remember if FB was previously on/off"
                    n554 = feedback #45(FALSE) -> (w1280:bool)
                    n555 = case shown="True" w1284 {
                      tunnel: [w1287 w1303] -> w1285
                      tunnel: "BD 2 Amplitude 3" -> [w1287 _]
                      tunnel: [FALSE TRUE] -> w1281
                      tunnel: w1280 -> [_ w1289]
                      frame False {
                      }
                      frame True {
                        # "Makes it so first time FB run when turned on, the PID sees the detector intensity from the last time FB was running, rather than something near zero. Especially assuming the setpoint is not changing, this will make the FB more stable when resuming, and not overshoot the turnon intensity."
                        # "FB output range: 0 should be low, full scale is 12 bits.\nBut be careful not to go over, then higher bits just get ignored by RF board, so output will actually jump down and be unstable. Keep it under 4000 to be safe."
                        n556 = local read "Green FB Sum"() -> (w1288:i16)
                        n557 = feedback-in #46(w1288) -> ()
                        n558 = feedback #46(i16 0 ("Green FB Sum")) -> (w1291:i16)
                        n559 = Select(t=w1288, s=w1289, f=w1291) -> (s? t:f=w1290:i16)
                        n560 = Bundle("P3 2"="P3 2", "I3 2"="I3 2", "D3 2"="D3 2") -> (w1302:cluster{"P3 2":i16, "I3 2":i16, "D3 2":i16})  [unwired: 1 in]
                        n561 = Bundle("RF synth green feedback max"="RF synth green feedback max", i16 0) -> (w1294:cluster{"RF synth green feedback max":i16, i16})  [unwired: 1 in]
                        n562 = call "Slower PID.vi"("process variable"=w1290, "reset?"="Green FB Reset 2", "setpoint"="Green FB Setpoint 2", "PID gains (x 2^8)"=w1302, "output range"=w1294) -> ("output"=w1304:i16)  [unwired: 10 out]
                        n563 = To Unsigned Word Integer(number=w1304) -> (unsigned 16bit integer=w1303:u16)
                      }
                    }
                    n564 = feedback-in #45(w1281) -> ()
                  }
                  frame Enabled {
                  }
                }
              }
            }
            n565 = Split Number(x=w845) -> (hi(x)=w844:u32, lo(x)=w843:u32)
            n566 = Boolean To (0,1)(Boolean="+ phase (DIO)") -> (0, 1=w805:i16)
            n567 = Split Number(x=w844) -> (lo(x)=w842:u16)  [unwired: 1 out]
            n568 = Split Number(x=w843) -> (hi(x)=w841:u16, lo(x)=w840:u16)
            n569 = Split Number(x=w842) -> (hi(x)=w834:u8, lo(x)=w833:u8)
            n570 = Split Number(x=w841) -> (hi(x)=w832:u8, lo(x)=w831:u8)
            n571 = Split Number(x=w840) -> (hi(x)=w830:u8, lo(x)=w829:u8)
            n572 = Multiply(x=w805, y="Phase count adjustment (DIO)") -> (x*y=w801:i16)
            n573 = feedback #47(TRUE) -> (w790:bool)
            n574 = Not(x=w790) -> (.not. x?=w789:bool)
            n575 = feedback-in #47(w789) -> ()
            n576 = feedback #48(i16 0) -> (w803:i16)
            n577 = Subtract(x=w803, y=w801) -> (x-y=w802:i16)
            "DIO Relative phase" <- w802
            n578 = feedback-in #48(w802) -> ()
            n579 = Add(x=w808, y=w801) -> (x+y=w807:u32)
            n580 = Build Array "BD 1 nu Stack"(w834, w833, w832, w831, w830, w829) -> (w828:u8[])
            n581 = Not Equal?(x=w768, y=u8 3) -> (x != y?=w777:bool)
            n582 = case "Store in RF board F1 or F2" shown="True" w789 {
              tunnel: [w1000 w1004] -> w819
              tunnel: [u8 10 u8 4] -> w820
              tunnel: "Swap F1 and F2" -> [w1001 w1004]
              tunnel: "BD 2 Frequency 1" -> [_ w1003]
              tunnel: "BD 2 Frequency 2" -> [w999 _]
              tunnel: [w999 w1003] -> w785
              frame False {
                # "for RF synth controls\ngreen: F1/F2 stay same"
                # "F2 address (hex)"
                n583 = Not(x=w1001) -> (.not. x?=w1000:bool)
              }
              frame True {
                # "low chooses F1"
                # "F1 address (hex)"
              }
            }
            n584 = Select(t=w785, s="RF synth bd controls green", f=w784) -> (s? t:f=w783:u64)
            n585 = Split Number(x=w783) -> (hi(x)=w839:u32, lo(x)=w838:u32)
            n586 = Split Number(x=w839) -> (lo(x)=w837:u16)  [unwired: 1 out]
            n587 = Split Number(x=w838) -> (hi(x)=w836:u16, lo(x)=w835:u16)
            n588 = Split Number(x=w837) -> (hi(x)=w827:u8, lo(x)=w826:u8)
            n589 = Split Number(x=w836) -> (hi(x)=w825:u8, lo(x)=w824:u8)
            n590 = Split Number(x=w835) -> (hi(x)=w823:u8, lo(x)=w822:u8)
            n591 = feedback #49(u16 0 ("BD 2 Amplitude 3")) -> (w774:u16)
            n592 = Select(t=w774, s=w777, f=w776) -> (s? t:f=w775:u16)
            n593 = feedback-in #49(w775) -> ()
            n594 = And(x=w777, y=w780) -> (x .and. y?=w779:bool)
            n595 = Build Array "BD 2 nu Stack"(w827, w826, w825, w824, w823, w822) -> (w821:u8[])
            n596 = Select(t=w774, s=w779, f=w776) -> (s? t:f=w757:u16)
            n597 = flat-sequence "Update trap RF synth board settings to be used for the upcoming trap cycle." {
              tunnel: w821 -> [w948]
              tunnel: w828 -> [w949]
              tunnel: [w949] -> w772
              tunnel: [w948] -> w771
              tunnel: w820 -> [w950]
              tunnel: w772 -> [w952]
              tunnel: w771 -> [w951]
              tunnel: w759 -> [w963]
              tunnel: w761 -> [w962]
              tunnel: w760 -> [w961]
              frame #0 {
                # "To possibly delay\nthese writes to very\nend of loop (for x and\ny phase adjust)"
                n598 = call "Wait8"("Count(Ticks)"="Next trap write delay (ticks)") -> ()  [unwired: 1 out]
              }
              frame #1 {
                # "Next trap RF frequency:\n\nWrite next trap cycle frequency to buffer."
                n599 = for {
                  tunnel: w952 -> [w958] mode=indexing
                  tunnel: w951 -> [w957] mode=indexing
                  tunnel: w950 -> [w955]
                  i -> [w956]
                  n600 = To Unsigned Byte Integer(number=w956) -> (unsigned 8bit integer=w953:u8)
                  n601 = Add(x=w955, y=w953) -> (x+y=w954:u8)
                  n602 = call "write to RF synth bd.vi"("Address Byte"=w954, "BD 2 Byte"=w957, "BD 1 Byte"=w958) -> ()
                }
              }
              frame #2 {
                w959 = TRUE ("Connector1/DIO15")
                # "Send udclk high\n(BD 1 and 2) to make the new frequency active in F1 or F2 word. But it won't actually be the used frequency until FSK switches to it (begining of next cycle)."
                n603 = xnode "FPGA I/O Node"("Connector1/DIO30"=w959, "Connector1/DIO29"=w959) -> ()  [unwired: 2 in, 2 out]
              }
              frame #3 {
                w960 = FALSE ("Connector1/DIO15")
                n604 = xnode "FPGA I/O Node"("Connector1/DIO30"=w960, "Connector1/DIO29"=w960) -> ()  [unwired: 2 in, 2 out]
              }
              frame #4 {
                # "Next trap RF phase offset:\n\nSet the next trap cycle amplitude to the buffer. Won't become active until udclk is set high at proper time at the begining of the next cycle."
                n605 = case shown="True" w963 {
                  tunnel: w962 -> [_ w964]
                  tunnel: w961 -> [_ w965]
                  frame False {
                  }
                  frame True {
                    # "phase 1 address start"
                    n606 = for {
                      tunnel: w964 -> [w972] mode=indexing
                      tunnel: w965 -> [w971] mode=indexing
                      tunnel: u8 0 -> [w969]
                      i -> [w970]
                      n607 = To Unsigned Byte Integer(number=w970) -> (unsigned 8bit integer=w967:u8)
                      n608 = Add(x=w969, y=w967) -> (x+y=w968:u8)
                      n609 = call "write to RF synth bd.vi"("Address Byte"=w968, "BD 2 Byte"=w971, "BD 1 Byte"=w972) -> ()
                    }
                  }
                }
              }
              frame #5 {
                # "Prep to reset RF phase to zero at start of next cycle. Only reset BD 1. Do nothing to BD 2. This puts the settings in the buffer. A udclk high will make both this phase reset and possibly a new phase offset setting active."
                n610 = case shown="True" "RF phase reset before cycles" {
                  frame False {
                  }
                  frame True {
                    w975 = u8 66  # BD 1 reset
                    n611 = call "write to RF synth bd.vi"("Address Byte"=u8 31, "BD 2 Byte"=u8 2, "BD 1 Byte"=w975) -> ()
                  }
                }
              }
              frame #6 {
                # "Address"
                # "Data BD 2"
                # "Data BD 1"
                # "If phase reset wasn't chosen previously, these actions will have no affect. For both BD's, data should be binary 10, and address should be hex 1F (bin 01 1111)"
                # "This sets up the digital communication lines to restart phase accumulation (start RF running agin). It cancels out the possible phase reset. Just need to set WR DIO low then udclk DIOhigh  to make this happen. Doing this here early (and not using the usual board write function) speeds things up.\n\nRestarts RF (BD 1 only, BD2 never stopped in first place)."
                n612 = xnode "FPGA I/O Node"("Connector1/DIO0"=FALSE, "Connector1/DIO1"=FALSE, "Connector1/DIO2"=FALSE, "Connector1/DIO3"=FALSE, "Connector1/DIO4"=FALSE, "Connector1/DIO5"=FALSE, "Connector1/DIO6"=TRUE, "Connector1/DIO7"=FALSE, "Connector1/DIO8"=FALSE, "Connector1/DIO9"=TRUE, "Connector1/DIO10"=TRUE, "Connector1/DIO11"=TRUE, "Connector1/DIO12"=TRUE, "Connector1/DIO13"=TRUE, "Connector1/DIO20"=FALSE, "Connector1/DIO21"=FALSE, "Connector1/DIO22"=FALSE, "Connector1/DIO23"=FALSE, "Connector1/DIO24"=FALSE, "Connector1/DIO25"=FALSE, "Connector1/DIO26"=TRUE, "Connector1/DIO27"=FALSE) -> ()  [unwired: 22 in, 22 out]
              }
            }
            n613 = feedback #50(fxp<+,8,8> 0.0) -> (w754:fxp<+,8,8>)
            n614 = Increment(x=w754) -> (x+1=w752:fxp<+,8,8>)
            n615 = feedback-in #50(w752) -> ()
            n616 = case "Trap RF phase offset control methods" shown="3" "Phase offset method" {
              tunnel: [fxp<+,14,14> 0.0 ("Phase BD 1") w898 w913 w942] -> w762
              tunnel: "Phase Trap 1" -> [_ w899 w914 _]
              tunnel: w768 -> [_ w900 w915 w943]
              tunnel: [FALSE TRUE TRUE TRUE] -> w759
              tunnel: "Phase Trap 2" -> [_ w896 w911 _]
              tunnel: w752 -> [_ _ w910 _]
              frame 0, Default {
              }
              frame 1 {
                # "Constant increment of phase offset with each trap cycle. This results in a constant phase difference between trap cycles. \nOnly for traps 1 and 2 (set phase offset to zero for set three)."
                n617 = case shown="1, Default" w900 {
                  tunnel: w899 -> [_ _ w906]
                  tunnel: [w902 fxp<+,14,14> 0.0 w907] -> w898
                  tunnel: w896 -> [w901 _ _]
                  frame 2 {
                    n618 = feedback #51(fxp<+,14,14> 0.0) -> (w904:fxp<+,14,14>)
                    n619 = Add(x=w901, y=w904) -> (x+y=w902:fxp<+,14,14>)
                    n620 = feedback-in #51(w902) -> ()
                  }
                  frame 3 {
                  }
                  frame 1, Default {
                    n621 = feedback #52(fxp<+,14,14> 0.0) -> (w909:fxp<+,14,14>)
                    n622 = Add(x=w906, y=w909) -> (x+y=w907:fxp<+,14,14>)
                    n623 = feedback-in #52(w907) -> ()
                  }
                }
              }
              frame 2 {
                # "Changing increment of phase offset with each trap cycle. This results in a constant change in phase difference between trap cycles. \nOnly for traps 1 and 2 (set phase offset to zero for set three)."
                n624 = case shown="2" w915 {
                  tunnel: w914 -> [_ _ w925]
                  tunnel: [w916 fxp<+,14,14> 0.0 w923] -> w913
                  tunnel: w911 -> [w918 _ _]
                  tunnel: w910 -> [w919 _ w926]
                  frame 2 {
                    n625 = Multiply(x=w918, y=w919) -> (x*y=w917:fxp<+,16,16>)
                    n626 = feedback #53(fxp<+,14,14> 0.0) -> (w921:fxp<+,14,14>)
                    n627 = Add(x=w917, y=w921) -> (x+y=w916:fxp<+,14,14>)
                    n628 = feedback-in #53(w916) -> ()
                  }
                  frame 3 {
                  }
                  frame 1, Default {
                    n629 = Multiply(x=w925, y=w926) -> (x*y=w924:fxp<+,16,16>)
                    n630 = feedback #54(fxp<+,14,14> 0.0) -> (w928:fxp<+,14,14>)
                    n631 = Add(x=w924, y=w928) -> (x+y=w923:fxp<+,14,14>)
                    n632 = feedback-in #54(w923) -> ()
                  }
                }
              }
              frame 3 {
                w935 = u32 1013904223  # LCG constant C (add)
                w937 = fxp<+,21,21> 1664525.0  # LCG constant A (multiply)
                # "Set a random phase offset. Random number generated using the LCG method. Constants and method taken from NI white noise generator code (method is general though)."
                # "shift to 14 significant bits"
                n633 = feedback #55(u32 4294967295 ("seed")) -> (w932:u32)
                n634 = Multiply(x=w932, y=w937) -> (x*y=w936:u32)
                n635 = Split Number(x=w932) -> (hi(x)=w938:u16)  [unwired: 1 out]
                n636 = To Unsigned Word Integer(number=w938) -> (unsigned 16bit integer=w930:u16)
                n637 = Add(x=w936, y=w935) -> (x+y=w934:fxp<+,32,32>)
                n638 = To Unsigned Long Integer(number=w934) -> (unsigned 32bit integer=w931:u32)
                n639 = feedback-in #55(w931) -> ()
                n640 = Scale By Power Of 2(n=i8 -2 ("Uniform scale factor"), x=w930) -> (x*2^n=w939:u16)
                n641 = To Fixed-Point(number=w939) -> (fixed-point=w929:fxp<+,14,14>)  [unwired: 1 in]
                "Random phase generated" <- w929
                n642 = case shown="1, Default" w943 {
                  tunnel: [w944 fxp<+,14,14> 0.0 w946] -> w942
                  tunnel: w929 -> [w944 _ w946]
                  frame 2 {
                  }
                  frame 3 {
                  }
                  frame 1, Default {
                  }
                }
              }
            }
            n643 = To Unsigned Word Integer(number=w762) -> (unsigned 16bit integer=w767:u16)
            n644 = Split Number(x=w767) -> (hi(x)=w765:u8, lo(x)=w766:u8)
            n645 = Split Number(x=u16 0) -> (hi(x)=w763:u8, lo(x)=w764:u8)
            n646 = Build Array ("BD 1 A Stack")(w765, w766) -> (w761:u8[])
            n647 = Build Array ("BD 1 A Stack")(w763, w764) -> (w760:u8[])
          }
        }
      }
    }
  }
  n648 = while "532 nm green fluorescent laser interlacing (DO to IA 532 nm AOM ME amp)." {
    shift-right: [w1308] -> _
    shift-left: w2 -> [w1313]
    shift-right: [w1307] -> _
    shift-left: w3 -> [w1305]
    stop <- FALSE stop-if-true
    n649 = flat-sequence {
      tunnel: w1313 -> [w1316]
      tunnel: [w1315] -> w1311
      tunnel: [w1316] -> w1309
      tunnel: [w1317] -> w1306
      tunnel: w1305 -> [w1317]
      tunnel: [w1320] -> w1312
      tunnel: w1311 -> [w1320]
      tunnel: [w1319] -> w1310
      tunnel: w1309 -> [w1319]
      tunnel: w1306 -> [w1318]
      tunnel: [w1329] -> w1308
      tunnel: w1312 -> [w1349]
      tunnel: w1310 -> [w1346]
      tunnel: [w1338] -> w1307
      frame #0 {
        n650 = call "Loop Timer9"("Count(Ticks)"=w1316) -> ("Tick Count(Ticks)"=w1315:u32)
      }
      frame #1 {
        # "Then to PRL 440 amp\nOR to RF synth board FSK in"
        n651 = xnode "FPGA I/O Node"("Connector1/DIO37"=w1318, "Connector1/DIO38"=w1318, "Connector1/DIO39"=w1318, "Connector1/DIO26"=w1318, "Connector1/DIO27"=w1318, "Connector1/DIO32"=w1318) -> ()  [unwired: 6 in, 6 out]
      }
      frame #2 {
        n652 = feedback-in #56(w1349) -> ()
        n653 = feedback #56(w1349) -> (w1348:u32)
        n654 = Subtract(x=w1349, y=w1348) -> (x-y=w1347:u32)
        n655 = Subtract(x=w1347, y=w1346) -> (x-y=w1322:u32)
        n656 = Number To Boolean Array(number=w1322) -> (Boolean array=w1323:bool[])
        n657 = Or Array Elements(Boolean array=w1323) -> (logical OR=w1321:bool)
        n658 = Boolean To (0,1)(Boolean="+ phase (GI)") -> (0, 1=w1334:i16)
        n659 = Multiply(x=w1334, y="Phase count adjustment (GI)") -> (x*y=w1331:i16)
        n660 = Boolean To (0,1)(Boolean=w1321) -> (0, 1=w1328:i16)
        n661 = To Unsigned Byte Integer(number=w1328) -> (unsigned 8bit integer=w1325:u8)
        n662 = feedback #57(i16 0) -> (w1332:i16)
        n663 = feedback #58(u8 0) -> (w1326:u8)
        n664 = Add(x=w1325, y=w1326) -> (x+y=w1324:u8)
        "GI Late Counter" <- w1324
        n665 = feedback-in #58(w1324) -> ()
        n666 = Subtract(x=w1332, y=w1331) -> (x-y=w1330:i16)
        "GI Relative phase" <- w1330
        n667 = feedback-in #57(w1330) -> ()
        n668 = feedback #59(TRUE) -> (w1341:bool)
        n669 = case shown="0, Default" "Operating Mode" {
          tunnel: [TRUE FALSE w1355] -> w1338
          tunnel: w1341 -> [_ _ w1352]
          frame 0, Default {
          }
          frame 1 {
          }
          frame 2 {
            n670 = Not(x=w1352) -> (.not. x?=w1354:bool)
            n671 = Select(t=w1354, s="Invert GI", f=w1352) -> (s? t:f=w1355:bool)
          }
        }
        n672 = Not(x=w1341) -> (.not. x?=w1337:bool)
        n673 = Select(t="Green interlace ON count", s=w1337, f="Green interlace OFF count") -> (s? t:f=w1343:u16)
        n674 = Subtract(x=w1343, y=w1322) -> (x-y=w1335:u32)
        n675 = Add(x=w1335, y=w1331) -> (x+y=w1329:u32)
        n676 = feedback-in #59(w1337) -> ()
      }
    }
  }
  n677 = while "Green excitation laser feedback measurement" {
    shift-right: [w1356] -> _
    shift-left: w2 -> [w1361]
    stop <- FALSE stop-if-true
    n678 = flat-sequence {
      tunnel: w1361 -> [w1363]
      tunnel: [w1364] -> w1359
      tunnel: [w1363] -> w1357
      tunnel: [w1371] -> w1360
      tunnel: w1359 -> [w1371]
      tunnel: [w1370] -> w1358
      tunnel: w1357 -> [w1370]
      tunnel: [w1383] -> w1356
      tunnel: w1360 -> [w1394]
      tunnel: w1358 -> [w1391]
      frame #0 {
        n679 = call "Loop Timer6"("Count(Ticks)"=w1363) -> ("Tick Count(Ticks)"=w1364:u32)
      }
      frame #1 {
        n680 = xnode "FPGA I/O Node"("Connector1/DIO35"=TRUE) -> ("Chassis2/Mod2/AI0"=w1369:i16, "Chassis2/Mod2/AI1"=w1368:i16, "Chassis2/Mod2/AI2"=w1365:i16)  [unwired: 4 in, 4 out]
        "Green FB Sum" <- w1365
        n681 = Bundle("Chassis2/Mod2/AI0"=w1369, "Chassis2/Mod2/AI1"=w1368, "Chassis2/Mod2/AI2"=w1365) -> (→"Green FB Signals":T10)  [unwired: 1 out]
      }
      frame #2 {
        n682 = feedback-in #60(w1394) -> ()
        n683 = feedback #60(w1394) -> (w1393:u32)
        n684 = Subtract(x=w1394, y=w1393) -> (x-y=w1392:u32)
        n685 = xnode "FPGA I/O Node"("Connector1/DIO35"=FALSE) -> ()  [unwired: 1 in, 1 out]
        n686 = Subtract(x=w1392, y=w1391) -> (x-y=w1373:u32)
        n687 = Subtract(x="Green FB Count", y=w1373) -> (x-y=w1387:u32)
        n688 = Number To Boolean Array(number=w1373) -> (Boolean array=w1374:bool[])
        n689 = Or Array Elements(Boolean array=w1374) -> (logical OR=w1372:bool)
        "Green FB Late?" <- w1372
        n690 = Boolean To (0,1)(Boolean="+ phase (Green FB)") -> (0, 1=w1385:i16)
        n691 = Boolean To (0,1)(Boolean=w1372) -> (0, 1=w1379:i16)
        n692 = Multiply(x=w1385, y="Phase count adjustment (Green FB)") -> (x*y=w1380:i16)
        n693 = Add(x=w1387, y=w1380) -> (x+y=w1383:u32)
        n694 = To Unsigned Word Integer(number=w1379) -> (unsigned 16bit integer=w1376:u16)
        n695 = feedback #61(i16 0) -> (w1382:i16)
        n696 = Subtract(x=w1382, y=w1380) -> (x-y=w1381:i16)
        "Green FB Relative Phase" <- w1381
        n697 = feedback-in #61(w1381) -> ()
        n698 = feedback #62(u16 0) -> (w1377:u16)
        n699 = Add(x=w1376, y=w1377) -> (x+y=w1375:u16)
        "Green Late Counter" <- w1375
        n700 = feedback-in #62(w1375) -> ()
      }
    }
  }
  n701 = while "Control APD data integration - stream to host" {
    shift-right: [w1397] -> _
    shift-left: w5 -> [w1402]
    stop <- FALSE stop-if-true
    n702 = flat-sequence {
      tunnel: w1402 -> [w1404]
      tunnel: [w1405] -> w1400
      tunnel: [w1404] -> w1398
      tunnel: [w1413] -> w1401
      tunnel: w1400 -> [w1413]
      tunnel: [w1412] -> w1399
      tunnel: w1398 -> [w1412]
      tunnel: [w1411] -> w1396
      tunnel: [w1410] -> w1395
      tunnel: [w1447] -> w1397
      tunnel: w1401 -> [w1459]
      tunnel: w1399 -> [w1456]
      tunnel: w1396 -> [w1440]
      tunnel: w1395 -> [w1439]
      frame #0 {
        n703 = call "Loop Timer4"("Count(Ticks)"=w1404) -> ("Tick Count(Ticks)"=w1405:u32)
      }
      frame #1 {
        n704 = flat-sequence {
          tunnel: [w1415] -> w1409
          tunnel: w1409 -> [w1417]
          tunnel: [w1419] -> w1408
          tunnel: [w1418] -> w1407
          tunnel: [w1417] -> w1406
          tunnel: [w1425] -> w1410
          tunnel: [w1426] -> w1411
          tunnel: w1408 -> [w1426]
          tunnel: w1407 -> [w1425]
          tunnel: w1406 -> [w1424]
          frame #0 {
            # "use two separate variable so each APD won't\nhave to wait to read"
            n705 = feedback #63(FALSE) -> (w1414:bool)
            "APD1 out state" <- w1414
            "APD2 out state" <- w1414
            n706 = Not(x=w1414) -> (.not. x?=w1415:bool)
            n707 = feedback-in #63(w1415) -> ()
          }
          frame #1 {
            n708 = local read "APD 1 Counts 1"() -> (w1423:u32)
            n709 = local read "APD 1 Counts 0"() -> (w1422:u32)
            n710 = local read "APD 2 Counts 1"() -> (w1421:u32)
            n711 = local read "APD 2 Counts 0"() -> (w1420:u32)
            n712 = Select(t=w1423, s=w1417, f=w1422) -> (s? t:f=w1419:u32)
            n713 = Select(t=w1421, s=w1417, f=w1420) -> (s? t:f=w1418:u32)
          }
          frame #2 {
            n714 = case shown="True" w1424 {
              frame False {
                w1427 = u32 0 ("APD 1 Counts 0")
                n715 = local write "APD 1 Counts 0"(w1427) -> ()
                n716 = local write "APD 2 Counts 0"(w1427) -> ()
              }
              frame True {
                w1428 = u32 0 ("APD 1 Counts 1")
                n717 = local write "APD 1 Counts 1"(w1428) -> ()
                n718 = local write "APD 2 Counts 1"(w1428) -> ()
              }
            }
          }
        }
      }
      frame #2 {
        n719 = feedback-in #64(w1459) -> ()
        n720 = feedback #64(w1459) -> (w1458:u32)
        n721 = Subtract(x=w1459, y=w1458) -> (x-y=w1457:u32)
        n722 = Subtract(x=w1457, y=w1456) -> (x-y=w1432:u32)
        n723 = case shown="True" "APD to FIFO" {
          tunnel: w1440 -> [_ w1462]
          tunnel: w1439 -> [_ w1460]
          frame False {
          }
          frame True {
            n724 = flat-sequence {
              tunnel: 0 ("Timeout") -> [w1464]
              tunnel: w1462 -> [w1465]
              tunnel: [w1464] -> w1461
              tunnel: w1461 -> [w1467]
              tunnel: w1460 -> [w1466]
              frame #0 {
                n725 = xnode ("FIFO Write")("Element"=w1465, "Timeout"=w1464) -> ()  [unwired: 1 in, 2 out]
              }
              frame #1 {
                n726 = xnode ("FIFO Write")("Element"=w1466, "Timeout"=w1467) -> ()  [unwired: 1 in, 2 out]
              }
            }
          }
        }
        n727 = Subtract(x="APD Acq Rate Count", y=w1432) -> (x-y=w1448:u32)
        n728 = Number To Boolean Array(number=w1432) -> (Boolean array=w1433:bool[])
        n729 = Or Array Elements(Boolean array=w1433) -> (logical OR=w1431:bool)
        "APD Acq Late?" <- w1431
        n730 = Boolean To (0,1)(Boolean=w1431) -> (0, 1=w1438:i16)
        n731 = To Unsigned Word Integer(number=w1438) -> (unsigned 16bit integer=w1435:u16)
        n732 = Boolean To (0,1)(Boolean="+ phase (APD Acq)") -> (0, 1=w1444:i16)
        n733 = feedback #65(u16 0) -> (w1436:u16)
        n734 = Add(x=w1435, y=w1436) -> (x+y=w1434:u16)
        "APD Acq Late Counter" <- w1434
        n735 = feedback-in #65(w1434) -> ()
        n736 = Multiply(x=w1444, y="Phase Count Adjustment (APD Acq)") -> (x*y=w1441:i16)
        n737 = Add(x=w1448, y=w1441) -> (x+y=w1447:u32)
        n738 = feedback #66(i16 0) -> (w1446:i16)
        n739 = Subtract(x=w1446, y=w1441) -> (x-y=w1443:i16)
        "APD Acq Relative Phase" <- w1443
        n740 = feedback-in #66(w1443) -> ()
        n741 = To Word Integer(number=w1440) -> (16bit integer=w1449:i16)
        n742 = To Word Integer(number=w1439) -> (16bit integer=w1450:i16)
        n743 = Multiply(x="APD 1 AO scale factor", y=w1449) -> (x*y=w1430:i16)
        n744 = Multiply(x="APD 2 AO scale factor", y=w1450) -> (x*y=w1429:i16)
        n745 = xnode "FPGA I/O Node"("Connector0/AO6"=w1430, "Connector0/AO7"=w1429) -> ()  [unwired: 2 in, 2 out]
      }
    }
  }
  n746 = disable-structure shown="Disabled" {
    disable-tunnel: w2 -> [w1468 _]
    frame Disabled {
      n747 = while "APD 3 Counter" {
        tunnel: w1468 -> [_]
        stop <- FALSE stop-if-true
        n748 = flat-sequence {
          frame #0 {
            n749 = xnode "FPGA I/O Method Node"("FPGA I/O In"=refnum<k21> "Connector0/DIO12" ("APD 2 DO"), "Timeout"=-1) -> ()  [unwired: 2 out]
          }
          frame #1 {
            n750 = local read "APD3 int gate"() -> (w1472:bool)
            n751 = case shown="True" w1472 {
              frame False {
              }
              frame True {
                n752 = local read item#-1() -> (w1473)
                n753 = case shown="True" w1473 {
                  frame False {
                    n754 = local read "APD 3 Counts 0"() -> (w1475:u32)
                    n755 = Increment(x=w1475) -> (x+1=→"APD 3 Counts 0":u32)
                  }
                  frame True {
                    n756 = local read "APD 3 Counts 1"() -> (w1477:u32)
                    n757 = Increment(x=w1477) -> (x+1=→"APD 3 Counts 1":u32)
                  }
                }
              }
            }
          }
        }
      }
    }
    frame Enabled {
    }
  }
  n758 = disable-structure shown="Disabled" {
    disable-tunnel: w2 -> [w1479 _]
    disable-tunnel: w4 -> [w1478 _]
    frame Disabled {
      n759 = while "APD 3 Gating" {
        shift-right: [w1483] -> _
        shift-left: w1479 -> [w1488]
        shift-right: [w1482] -> _
        shift-left: w1478 -> [w1480]
        stop <- FALSE stop-if-true
        n760 = flat-sequence {
          tunnel: w1488 -> [w1491]
          tunnel: [w1490] -> w1486
          tunnel: [w1491] -> w1484
          tunnel: [w1492] -> w1481
          tunnel: w1480 -> [w1492]
          tunnel: [w1495] -> w1487
          tunnel: w1486 -> [w1495]
          tunnel: [w1494] -> w1485
          tunnel: w1484 -> [w1494]
          tunnel: w1481 -> [w1493]
          tunnel: [w1516] -> w1483
          tunnel: w1487 -> [w1527]
          tunnel: w1485 -> [w1524]
          tunnel: [w1496] -> w1482
          frame #0 {
            n761 = call "Loop Timer5"("Count(Ticks)"=w1491) -> ("Tick Count(Ticks)"=w1490:u32)
          }
          frame #1 {
            # "Signal maybe then sent through \na transistor before APD"
            n762 = xnode "FPGA I/O Node"("Connector0/DIO2"=w1493) -> ()  [unwired: 1 in, 1 out]
            "APD3 int gate" <- w1493
          }
          frame #2 {
            n763 = local read "APD Gate OFF Count"() -> (w1501:u16)
            n764 = local read "APD Gate ON Count"() -> (w1502:u16)
            n765 = feedback #67(TRUE) -> (w1521:bool)
            n766 = feedback-in #68(w1527) -> ()
            n767 = feedback #68(w1527) -> (w1526:u32)
            n768 = Not(x=w1521) -> (.not. x?=w1519:bool)
            n769 = feedback-in #67(w1519) -> ()
            n770 = Subtract(x=w1527, y=w1526) -> (x-y=w1525:u32)
            n771 = Select(t=w1502, s=w1519, f=w1501) -> (s? t:f=w1523:u16)
            n772 = Subtract(x=w1525, y=w1524) -> (x-y=w1504:u32)
            n773 = Subtract(x=w1523, y=w1504) -> (x-y=w1515:u32)
            n774 = Number To Boolean Array(number=w1504) -> (Boolean array=w1505:bool[])
            n775 = Or Array Elements(Boolean array=w1505) -> (logical OR=w1503:bool)
            n776 = Boolean To (0,1)(Boolean=w1503) -> (0, 1=w1510:i16)
            n777 = Boolean To (0,1)(Boolean="+ phase (APD 3 Gate)") -> (0, 1=w1513:i16)
            n778 = To Unsigned Byte Integer(number=w1510) -> (unsigned 8bit integer=w1507:u8)
            n779 = Multiply(x=w1513, y="Phase count adjustment (APD 3 Gate)") -> (x*y=w1511:i16)
            n780 = feedback #69(u8 0) -> (w1508:u8)
            n781 = Add(x=w1507, y=w1508) -> (x+y=w1506:u8)
            "APD 3 Gate Late Counter" <- w1506
            n782 = feedback-in #69(w1506) -> ()
            n783 = Add(x=w1515, y=w1511) -> (x+y=w1516:u32)
            n784 = feedback #70(i16 0) -> (w1518:i16)
            n785 = Subtract(x=w1518, y=w1511) -> (x-y=w1517:i16)
            "APD 3 Gate Relative Phase" <- w1517
            n786 = feedback-in #70(w1517) -> ()
            n787 = local read "APD Gate Operating Mode"() -> (w1500:u8)
            n788 = case shown="2" w1500 {
              tunnel: [TRUE FALSE w1530] -> w1497
              tunnel: w1521 -> [_ _ w1530]
              frame 0, Default {
              }
              frame 1 {
              }
              frame 2 {
              }
            }
            n789 = local read "Invert APD Gate"() -> (w1499:bool)
            n790 = Not(x=w1497) -> (.not. x?=w1498:bool)
            n791 = Select(t=w1498, s=w1499, f=w1497) -> (s? t:f=w1496:bool)
          }
        }
      }
    }
    frame Enabled {
    }
  }
  n792 = disable-structure shown="Disabled" {
    disable-tunnel: w2 -> [w1533 _]
    disable-tunnel: w3 -> [w1532 _]
    frame Disabled {
      n793 = while "633 nm red  fluorescent laser interlacing (DO to IA 633 nm AOM ME amp)." {
        shift-right: [w1654] -> _
        shift-left: w1533 -> [w1659]
        shift-right: [w1653] -> _
        shift-left: w1532 -> [w1651]
        stop <- FALSE stop-if-true
        n794 = flat-sequence {
          tunnel: w1659 -> [w1662]
          tunnel: [w1661] -> w1657
          tunnel: [w1662] -> w1655
          tunnel: [w1663] -> w1652
          tunnel: w1651 -> [w1663]
          tunnel: [w1666] -> w1658
          tunnel: w1657 -> [w1666]
          tunnel: [w1665] -> w1656
          tunnel: w1655 -> [w1665]
          tunnel: w1652 -> [w1664]
          tunnel: [w1675] -> w1654
          tunnel: w1658 -> [w1695]
          tunnel: w1656 -> [w1692]
          tunnel: [w1684] -> w1653
          frame #0 {
            n795 = call "Loop Timer8"("Count(Ticks)"=w1662) -> ("Tick Count(Ticks)"=w1661:u32)
          }
          frame #1 {
            # "Then to PRL 440 amp"
            n796 = xnode "FPGA I/O Node"("Connector1/DIO32"=w1664) -> ()  [unwired: 1 in, 1 out]
          }
          frame #2 {
            n797 = feedback-in #71(w1695) -> ()
            n798 = feedback #71(w1695) -> (w1694:u32)
            n799 = Subtract(x=w1695, y=w1694) -> (x-y=w1693:u32)
            n800 = Subtract(x=w1693, y=w1692) -> (x-y=w1668:u32)
            n801 = Number To Boolean Array(number=w1668) -> (Boolean array=w1669:bool[])
            n802 = Or Array Elements(Boolean array=w1669) -> (logical OR=w1667:bool)
            n803 = Boolean To (0,1)(Boolean="+ phase (RI)") -> (0, 1=w1680:i16)
            n804 = Multiply(x=w1680, y="Phase count adjustment (RI)") -> (x*y=w1677:i16)
            n805 = Boolean To (0,1)(Boolean=w1667) -> (0, 1=w1674:i16)
            n806 = To Unsigned Byte Integer(number=w1674) -> (unsigned 8bit integer=w1671:u8)
            n807 = feedback #72(i16 0) -> (w1678:i16)
            n808 = feedback #73(u8 0) -> (w1672:u8)
            n809 = Add(x=w1671, y=w1672) -> (x+y=w1670:u8)
            "RI Late Counter" <- w1670
            n810 = feedback-in #73(w1670) -> ()
            n811 = Subtract(x=w1678, y=w1677) -> (x-y=w1676:i16)
            "RI Relative phase" <- w1676
            n812 = feedback-in #72(w1676) -> ()
            n813 = feedback #74(TRUE) -> (w1687:bool)
            n814 = case shown="2" "Red Laser Operating Mode" {
              tunnel: [TRUE FALSE w1701] -> w1684
              tunnel: w1687 -> [_ _ w1698]
              frame 0, Default {
              }
              frame 1 {
              }
              frame 2 {
                n815 = Not(x=w1698) -> (.not. x?=w1700:bool)
                n816 = Select(t=w1700, s="Invert RI", f=w1698) -> (s? t:f=w1701:bool)
              }
            }
            n817 = Not(x=w1687) -> (.not. x?=w1683:bool)
            n818 = Select(t="Red interlace ON count", s=w1683, f="Red interlace OFF count") -> (s? t:f=w1689:u16)
            n819 = Subtract(x=w1689, y=w1668) -> (x-y=w1681:u32)
            n820 = Add(x=w1681, y=w1677) -> (x+y=w1675:u32)
            n821 = feedback-in #74(w1683) -> ()
          }
        }
      }
      n822 = while "473 nm blue  fluorescent laser interlacing (DO to blue laser digital control input)." {
        shift-right: [w1550] -> _
        shift-left: w1533 -> [w1553]
        shift-right: [w1549] -> _
        shift-left: w1532 -> [w1547]
        shift-right: [w1542] -> _
        shift-left: _ -> [w1541]
        shift-right: [w1534] -> _
        shift-left: u16 0 -> [w1537]
        stop <- FALSE stop-if-true
        n823 = flat-sequence {
          tunnel: w1553 -> [w1556]
          tunnel: [w1555] -> w1552
          tunnel: [w1556] -> w1551
          tunnel: [w1559] -> w1548
          tunnel: w1547 -> [w1559]
          tunnel: w1541 -> [w1558]
          tunnel: [w1558] -> w1540
          tunnel: [w1557] -> w1538
          tunnel: w1537 -> [w1557]
          tunnel: [w1564] -> w1546
          tunnel: w1552 -> [w1564]
          tunnel: [w1563] -> w1545
          tunnel: w1551 -> [w1563]
          tunnel: w1548 -> [w1562]
          tunnel: w1540 -> [w1561]
          tunnel: [w1561] -> w1539
          tunnel: w1538 -> [w1560]
          tunnel: [w1560] -> w1536
          tunnel: [w1569] -> w1544
          tunnel: [w1568] -> w1543
          tunnel: w1545 -> [w1568]
          tunnel: w1546 -> [w1569]
          tunnel: w1539 -> [w1567]
          tunnel: w1536 -> [w1566]
          tunnel: [w1565] -> w1535
          tunnel: [w1626] -> w1550
          tunnel: w1544 -> [w1644]
          tunnel: w1543 -> [w1641]
          tunnel: [w1614] -> w1549
          tunnel: [w1612] -> w1542
          tunnel: w1535 -> [w1609]
          tunnel: [w1610] -> w1534
          frame #0 {
            n824 = call "Loop Timer7"("Count(Ticks)"=w1556) -> ("Tick Count(Ticks)"=w1555:u32)
          }
          frame #1 {
            n825 = xnode "FPGA I/O Node"("Connector1/DIO28"=w1562) -> ()  [unwired: 1 in, 1 out]
          }
          frame #2 {
            n826 = case shown="True" w1567 {
              tunnel: w1566 -> [w1570 w1572]
              tunnel: [w1570 w1571] -> w1565
              frame False {
              }
              frame True {
                n827 = flat-sequence {
                  tunnel: [w1578] -> w1575
                  tunnel: [w1577] -> w1574
                  tunnel: [w1576] -> w1573
                  tunnel: w1572 -> [w1576]
                  tunnel: w1575 -> [w1595]
                  tunnel: w1574 -> [w1592]
                  tunnel: w1573 -> [w1594]
                  tunnel: [w1593] -> w1571
                  frame #0 {
                    # "5 ns timing resolution"
                    n828 = node-c288() -> (w1581:T7)  [unwired: 1 in]
                    n829 = timed-loop {
                      timing: w1581 -> [_]
                      timing-out: [_] -> w1580
                      tunnel: "Lifetime timeout APD1" -> [w1587]
                      tunnel: [w1582] -> w1577
                      tunnel: [w1583] -> w1578
                      i -> [w1584]
                      stop <- w1586 stop-if-true
                      n830 = xnode "FPGA I/O Node"() -> ("Connector0/DIO5"=w1585:bool)  [unwired: 1 in, 1 out]
                      n831 = To Unsigned Word Integer(number=w1584) -> (unsigned 16bit integer=w1582:u16)
                      n832 = Equal?(x=w1587, y=w1582) -> (x = y?=w1583:bool)
                      n833 = Or(x=w1585, y=w1583) -> (x .or. y?=w1586:bool)
                    }
                    n834 = node-c288(w1580) -> ()
                  }
                  frame #1 {
                    n835 = Not(x=w1595) -> (.not. x?=w1596:bool)
                    n836 = case shown="True" w1596 {
                      tunnel: w1592 -> [_ w1598]
                      tunnel: w1594 -> [w1597 w1600]
                      tunnel: [w1597 w1599] -> w1593
                      frame False {
                        # "timed out, do nothing"
                      }
                      frame True {
                        # "photon detected,record time"
                        n837 = case shown="True" "Lifetime to FIFO" {
                          tunnel: w1598 -> [_ w1606]
                          tunnel: w1600 -> [w1602 w1604]
                          tunnel: [w1602 w1603] -> w1599
                          frame False {
                            # "don't record time\n(can't if doing force feedback)"
                          }
                          frame True {
                            # "number of events in fifo"
                            n838 = xnode ("FIFO Method Node")("Element"=w1606, "Timeout"=0) -> ()  [unwired: 1 in, 2 out]
                            n839 = Increment(x=w1604) -> (x+1=w1603:u16)
                          }
                        }
                        "lifetime (ticks)" <- w1598
                      }
                    }
                  }
                }
              }
            }
          }
          frame #3 {
            # "Reading fifo is tricky here since\nunknown # of events"
            # "For lifetime measurement:\nInterlacing and pulse falling"
            n840 = feedback-in #75(w1644) -> ()
            n841 = feedback #75(w1644) -> (w1643:u32)
            n842 = Subtract(x=w1644, y=w1643) -> (x-y=w1642:u32)
            n843 = Subtract(x=w1642, y=w1641) -> (x-y=w1619:u32)
            n844 = Number To Boolean Array(number=w1619) -> (Boolean array=w1620:bool[])
            n845 = Or Array Elements(Boolean array=w1620) -> (logical OR=w1618:bool)
            n846 = Boolean To (0,1)(Boolean="+ phase (BI D)") -> (0, 1=w1631:i16)
            n847 = Multiply(x=w1631, y="Phase count adjustment (BI D)") -> (x*y=w1628:i16)
            n848 = Boolean To (0,1)(Boolean=w1618) -> (0, 1=w1625:i16)
            n849 = To Unsigned Byte Integer(number=w1625) -> (unsigned 8bit integer=w1622:u8)
            n850 = feedback #76(i16 0) -> (w1629:i16)
            n851 = feedback #77(u8 0) -> (w1623:u8)
            n852 = Add(x=w1622, y=w1623) -> (x+y=w1621:u8)
            "Blue Late Counter (D)" <- w1621
            n853 = feedback-in #77(w1621) -> ()
            n854 = Subtract(x=w1629, y=w1628) -> (x-y=w1627:i16)
            "BI Relative phase (D)" <- w1627
            n855 = feedback-in #76(w1627) -> ()
            n856 = feedback #78(TRUE) -> (w1636:bool)
            n857 = case shown="2" "Blue Laser Operating Mode (D)" {
              tunnel: [TRUE FALSE w1650] -> w1614
              tunnel: w1636 -> [_ _ w1647]
              frame 0, Default {
              }
              frame 1 {
              }
              frame 2 {
                n858 = Not(x=w1647) -> (.not. x?=w1649:bool)
                n859 = Select(t=w1649, s="Invert BI (D)", f=w1647) -> (s? t:f=w1650:bool)
              }
            }
            n860 = Subtract(x=w1609, y="Lifetime events to read blue") -> (x-y=w1607:u16)
            n861 = Not(x=w1636) -> (.not. x?=w1634:bool)
            n862 = Select(t="Blue interlace ON count (D)", s=w1634, f="Blue interlace OFF count (D)") -> (s? t:f=w1638:u16)
            n863 = Subtract(x=w1638, y=w1619) -> (x-y=w1632:u32)
            n864 = Add(x=w1632, y=w1628) -> (x+y=w1626:u32)
            n865 = feedback-in #78(w1634) -> ()
            n866 = Select(t=w1607, s="Lifetime read blue fifo", f=w1609) -> (s? t:f=w1610:u16)
            "lifetime events in fifo" <- w1610
            n867 = Equal?(x="Blue Laser Operating Mode (D)", y=u8 2) -> (x = y?=w1615:bool)
            n868 = Not(x=w1614) -> (.not. x?=w1613:bool)
            n869 = And(x=w1613, y=w1615) -> (x .and. y?=w1612:bool)
          }
        }
      }
    }
    frame Enabled {
    }
  }
